vi "32 Channel Model.vi"() -> ()   [LabVIEW 2018]
uses:
  <vilib>/Instr/_visa.llb/VISA Set IO Buffer Mask.ctl
  <vilib>/Instr/_visa.llb/VISA Configure Serial Port (Instr).vi
  <vilib>/Analysis/NI_AAL_SigProc.lvlib
panel:
  out "Difference Index":i32
  out "max difference":dbl
  out "C0 max value":dbl
  out "C0 index position":i32
  out "time in sec":u32
  out "Channel 33":i16[](graph)
  out "Channel 32":i16[](graph)
  out "C4  max value":dbl
  out "Ch4 index position":i32
  out "Channel 8 max":i32
  out "DIFFERENCE":dbl[](array[numeric])
  in  "?":bool
  in  "Select Channel 2":T1(ring)
  in  "Select Channel":T1(ring)
  out "Locations 28":dbl[](array[numeric])
  out "Locations C29":dbl[](array[numeric])
  out "Locations C30":dbl[](array[numeric])
  out "Locations C31":dbl[](array[numeric])
  out "Locations C24":dbl[](array[numeric])
  out "Locations 25":dbl[](array[numeric])
  out "Locations C26":dbl[](array[numeric])
  out "Locations C27":dbl[](array[numeric])
  out "Locations C20":dbl[](array[numeric])
  out "Locations C21":dbl[](array[numeric])
  out "Locations C22":dbl[](array[numeric])
  out "Locations C23":dbl[](array[numeric])
  out "Locations C16":dbl[](array[numeric])
  out "Locations C17":dbl[](array[numeric])
  out "Locations C18":dbl[](array[numeric])
  out "Locations C19":dbl[](array[numeric])
  out "Locations 12":dbl[](array[numeric])
  out "Locations 13":dbl[](array[numeric])
  out "Locations C14":dbl[](array[numeric])
  out "Locations C15":dbl[](array[numeric])
  out "Locations C8":dbl[](array[numeric])
  out "Locations C9":dbl[](array[numeric])
  out "Locations C10":dbl[](array[numeric])
  out "Locations C11":dbl[](array[numeric])
  out "Locations C4":dbl[](array[numeric])
  out "Locations C5":dbl[](array[numeric])
  out "Locations C6":dbl[](array[numeric])
  out "Locations C7":dbl[](array[numeric])
  out "Locations C3":dbl[](array[numeric])
  out "Locations C2":dbl[](array[numeric])
  out "Locations C1":dbl[](array[numeric])
  out "Locations C0":dbl[](array[numeric])
  in  "Infinite":bool
  in  "Stimulate":bool
  in  "Value 4":dbl=3.0 min=-10.0 max=10.0 step=0.01
  in  "Time 4":dbl=0.003 min=0.0001 max=60.0 step=1e-06
  in  "# of Pulse \n  Cycles":u16=24 min=1 step=1
  in  "Time 3":dbl=0.003 min=0.0001 max=60.0 step=1e-06
  in  "Value 3":dbl=-3.0 min=-10.0 max=10.0 step=0.01
  in  "Time 2":dbl=0.003 min=0.0001 max=60.0 step=1e-06
  in  "Value 2":dbl min=-10.0 max=10.0 step=0.01
  in  "# of Stimulation\n       Cycles":u16=1 min=1 max=65534 step=1
  in  "Time":dbl=0.9 min=0.0001 max=60.0 step=1e-06
  in  "Value":dbl min=-10.0 max=10.0 step=0.01
  in  "Stop Stimulation":bool
  in  "Channel Number":u8=1 max=31 step=1
  out "C31":bool
  out "C30":bool
  out "C29":bool
  out "C28":bool
  out "C27":bool
  out "C26":bool
  out "C25":bool
  out "C24":bool
  out "C20":bool
  out "C21":bool
  out "C22":bool
  out "C23":bool
  out "C19":bool
  out "C18":bool
  out "C17":bool
  out "C16":bool
  out "C15":bool
  out "C14":bool
  out "C13":bool
  out "C12":bool
  out "C8":bool
  out "C9":bool
  out "C10":bool
  out "C11":bool
  out "C4":bool
  out "C5":bool
  out "C6":bool
  out "C7":bool
  out "C0":bool
  out "C1":bool
  out "C2":bool
  out "C3":bool
  in  "?":bool
  out "?":bool
  out "Channel 31":i16[](graph)
  out "Channel 30":i16[](graph)
  out "Channel 29":i16[](graph)
  out "C28":u16
  out "C29":u16
  out "C30":u16
  out "C31":u16
  out "Channel 28":i16[](graph)
  out "Channel 27":i16[](graph)
  out "Channel 26":i16[](graph)
  out "Channel 25":i16[](graph)
  out "C27":u16
  out "C26":u16
  out "C25":u16
  out "C24":u16
  out "Channel 23":i16[](graph)
  out "Channel 22":i16[](graph)
  out "Channel 21":i16[](graph)
  out "C23":u16
  out "C22":u16
  out "C21":u16
  out "C20":u16
  out "Channel 20":i16[](graph)
  out "Channel 19":i16[](graph)
  out "Channel 18":i16[](graph)
  out "Channel 17":i16[](graph)
  out "C19":u16
  out "C18":u16
  out "C17":u16
  out "C16":u16
  out "Channel 16":i16[](graph)
  out "Channel 15":i16[](graph)
  out "Channel 14":i16[](graph)
  out "Channel 13":i16[](graph)
  out "C15":u16
  out "C14":u16
  out "C13":u16
  out "C12":u16
  out "Channel 12":i16[](graph)
  out "Channel 24":i16[](graph)
  out "Channel 11":i16[](graph)
  out "Channel 10":i16[](graph)
  out "Channel 9":i16[](graph)
  out "C11":u16
  out "C10":u16
  out "C9":u16
  out "C8":u16
  out "Channel 8":i16[](graph)
  out "C7":u16
  out "Channel 7":i16[](graph)
  out "C6":u16
  out "Channel 6":i16[](graph)
  out "C5":u16
  out "Channel 5":i16[](graph)
  out "C4":u16
  out "Channel 4":i16(graph)
  out "Channel 3":i16(graph)
  out "C3":u16
  out "C2":u16
  out "Channel 2":i16(graph)
  out "C1":u16
  out "Channel 1":i16(graph)
  out "Channel 0":i16(graph)
  out "C0":u16
  out "Ring 7":bool
  out "Ring 6":bool
  out "Ring 5":bool
  out "Ring 4":bool
  out "Ring 3":bool
  out "Ring 2":bool
  out "Ring 1":bool
  out "Ring 0":bool
  in  "VISA Stationary Port":refnum<visa-resource-name>
  # "Ring 0"
  # "Ring 0"
  # "Ring 1"
  # "Ring 2"
  # "Ring 1"
  # "Ring 3"
  # "Ring 4"
  # "Ring 5"
  # "Ring 7"
  # "Ring 6"
  # "Ring 2"
  # "Ring 3"
  # "Ring 4"
  # "Ring 5"
  # "Ring 6"
  # "Ring 7"
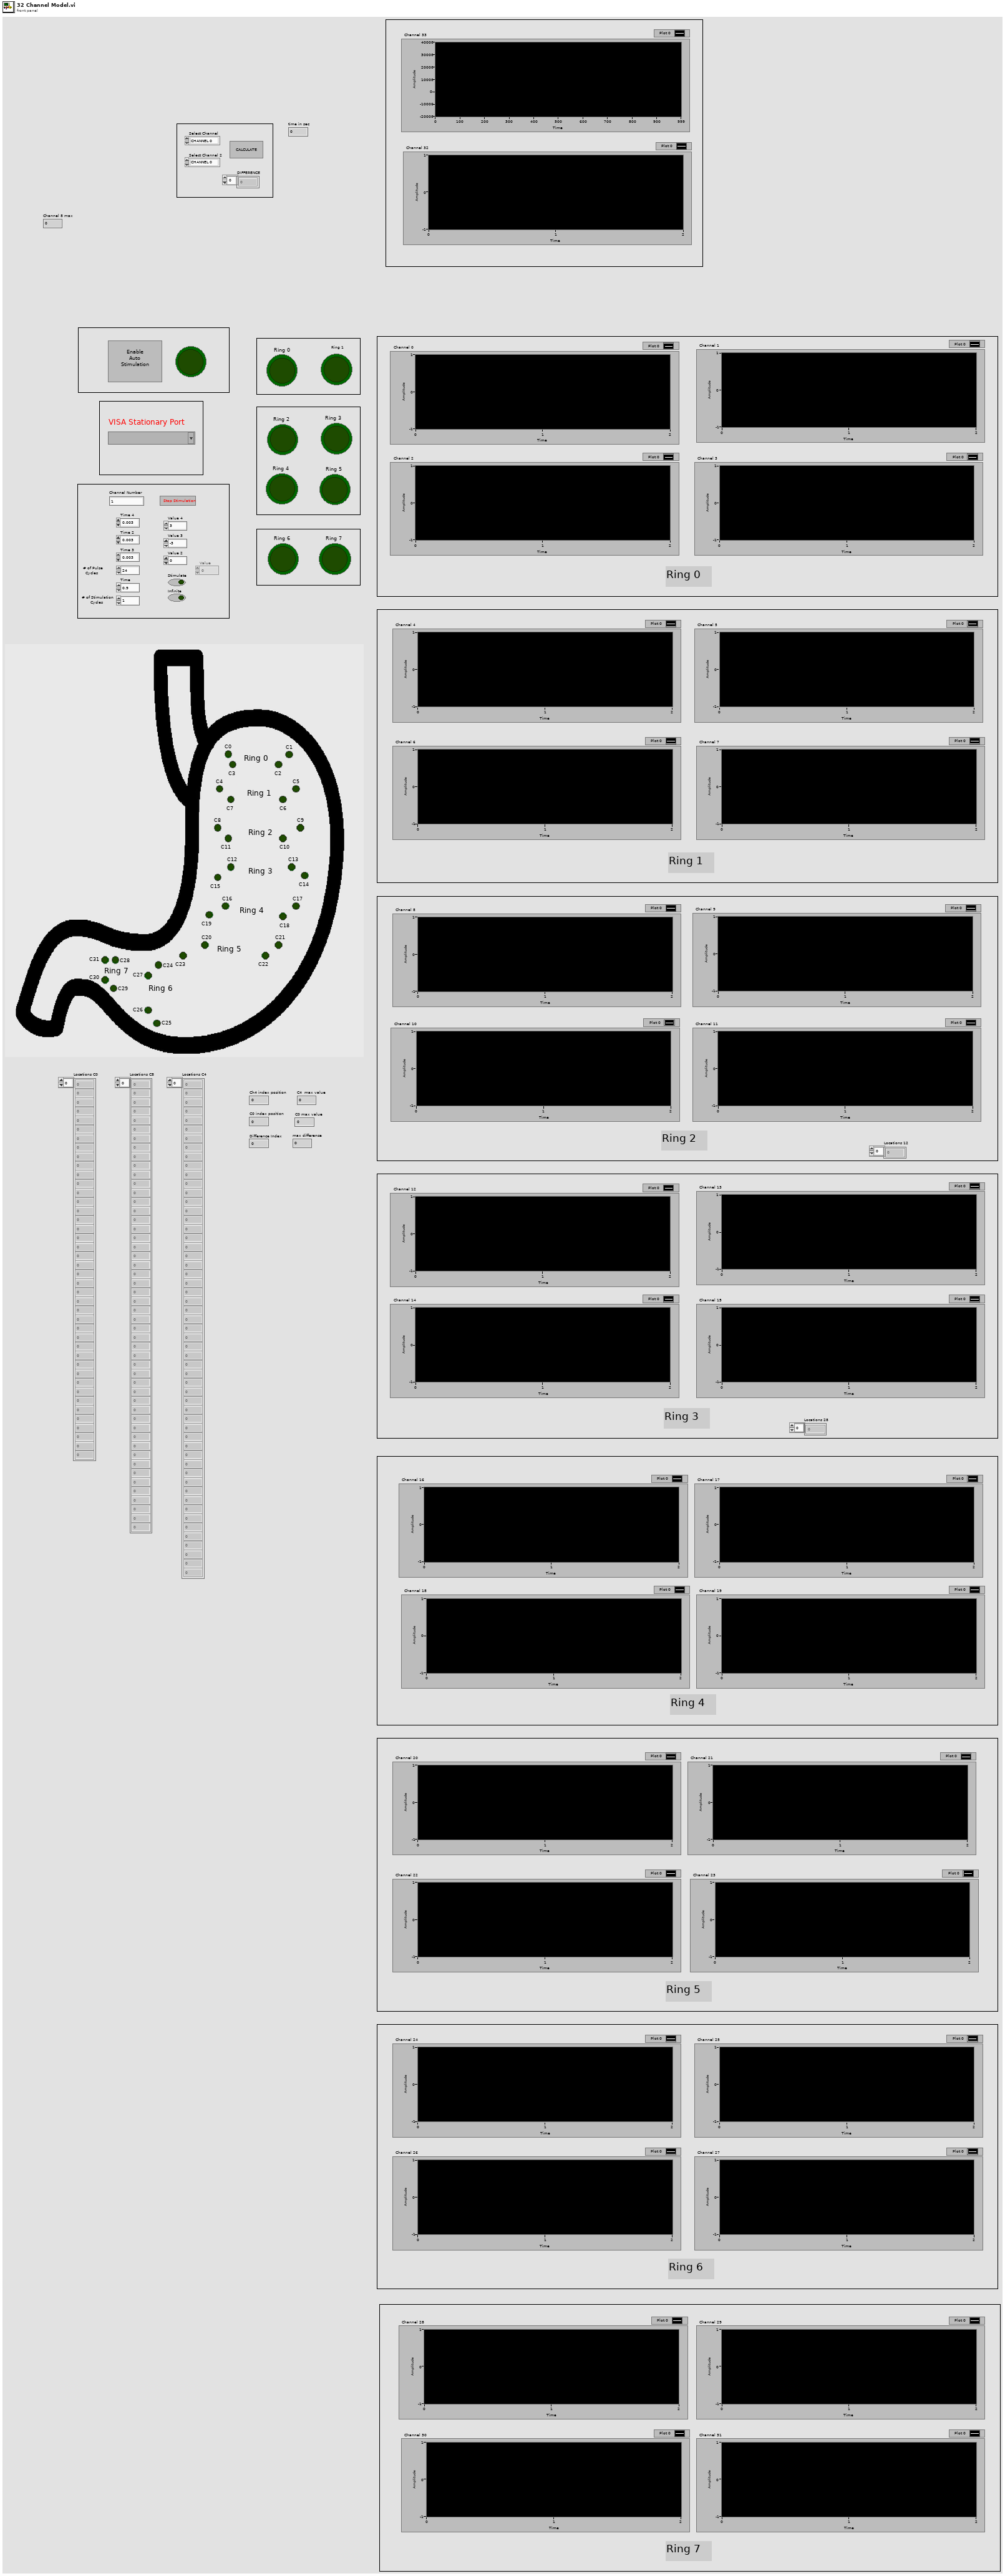
[diagram p1: front panel]
types:
  T1 = enum16{"CHANNEL 0", "CHANNEL 1", "CHANNEL 2 ", "CHANNEL 3 ", "CHANNEL 4 ", "CHANNEL 5 ", "CHANNEL 6", "CHANNEL  7", "CHANNEL 8 ", "CHANNEL 9", "CHANNEL 10", "CHANNEL 11", "CHANNEL 12", "CHANNEL 13", "CHANNEL 14", "CHANNEL 15", "CHANNEL 16", "CHANNEL 17", "CHANNEL 18", "CHANNEL 19", "CHANNEL 20", "CHANNEL 21", "CHANNEL 22", "CHANNEL 23", "CHANNEL 24", "CHANNEL 25", "CHANNEL 26", "CHANNEL 27", "CHANNEL 28", "CHANNEL 29", "CHANNEL 30", "CHANNEL 31"}
  T2 = typedef "VISA Set IO Buffer Mask.ctl" = u16
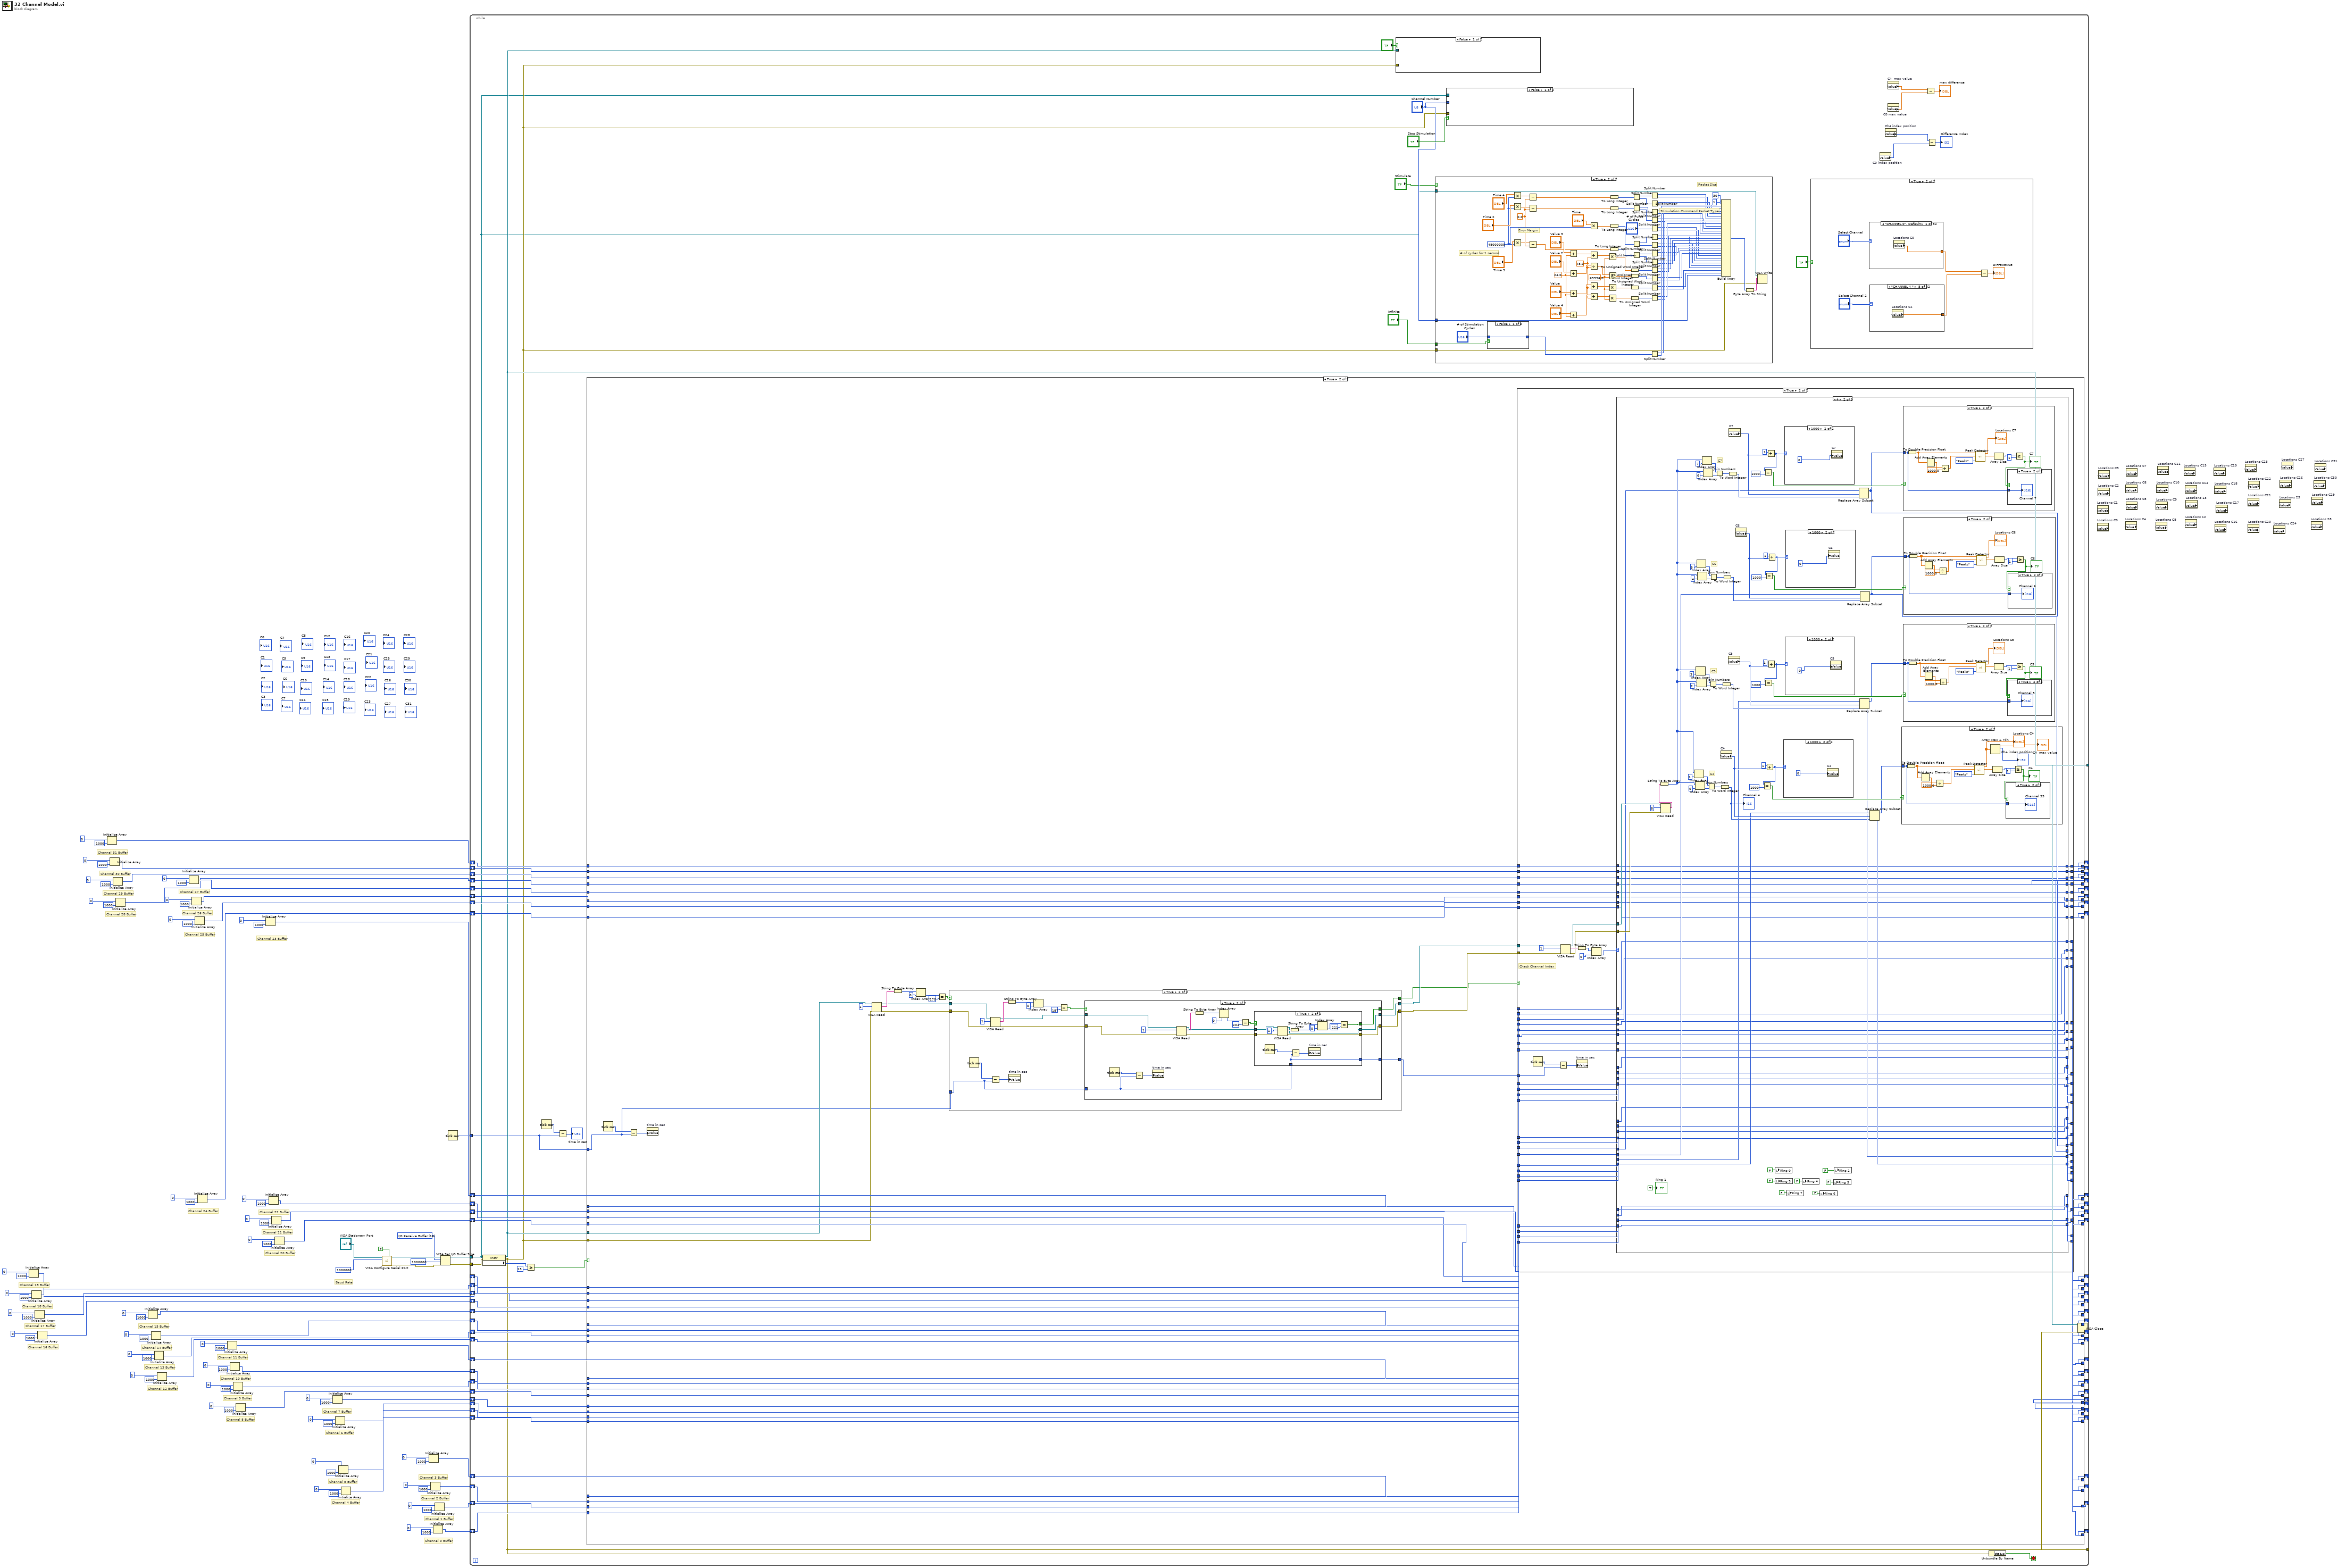
[diagram p0: block diagram]
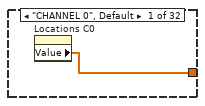
[diagram p3: hidden frame]
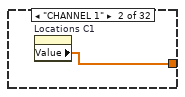
[diagram p4: hidden frame]
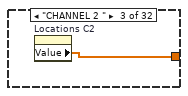
[diagram p5: hidden frame]
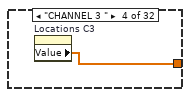
[diagram p6: hidden frame]
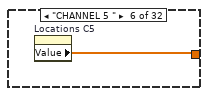
[diagram p7: hidden frame]
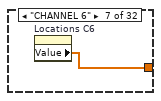
[diagram p8: hidden frame]
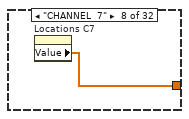
[diagram p9: hidden frame]
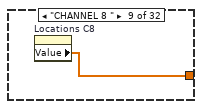
[diagram p10: hidden frame]
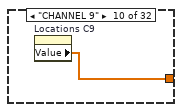
[diagram p11: hidden frame]
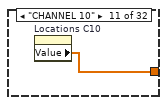
[diagram p12: hidden frame]
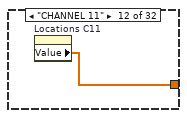
[diagram p13: hidden frame]
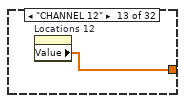
[diagram p14: hidden frame]
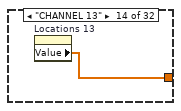
[diagram p15: hidden frame]
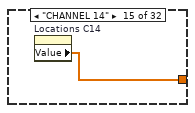
[diagram p16: hidden frame]
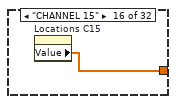
[diagram p17: hidden frame]
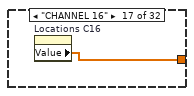
[diagram p18: hidden frame]
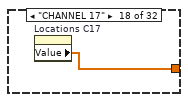
[diagram p19: hidden frame]
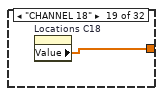
[diagram p20: hidden frame]
diagram:
  w104 = T2 16 items=["I/O Receive Buffer"=16, "I/O Transmit Buffer"=32, "I/O Receive and Transmit Buffer"=48] ("Mask")
  # "Channel 31 Buffer"
  # "Channel 30 Buffer"
  # "Channel 29 Buffer"
  # "Channel 28 Buffer"
  # "Channel 27 Buffer"
  # "Channel 26 Buffer"
  # "Channel 25 Buffer"
  # "Channel 24 Buffer"
  # "Channel 23 Buffer"
  # "Channel 22 Buffer"
  # "Channel 21 Buffer"
  # "Channel 20 Buffer"
  # "Channel 19 Buffer"
  # "Channel 18 Buffer"
  # "Channel 17 Buffer"
  # "Channel 16 Buffer"
  # "Channel 15 Buffer"
  # "Channel 14 Buffer"
  # "Channel 13 Buffer"
  # "Channel 12 Buffer"
  # "Channel 11 Buffer"
  # "Channel 10 Buffer"
  # "Channel 9 Buffer"
  # "Channel 8 Buffer"
  # "Channel 7 Buffer"
  # "Channel 6 Buffer"
  # "Channel 5 Buffer"
  # "Channel 4 Buffer"
  # "Channel 3 Buffer"
  # "Channel 2 Buffer"
  # "Channel 1 Buffer"
  # "Channel 0 Buffer"
  # "Baud Rate"
  n1 = Initialize Array(i16 0 ("element"), 1000 ("dimension size")) -> (w38:i16[])
  n2 = Initialize Array(i16 0 ("element"), 1000 ("dimension size")) -> (w39:i16[])
  n3 = Initialize Array(i16 0 ("element"), 1000 ("dimension size")) -> (w40:i16[])
  n4 = Initialize Array(i16 0 ("element"), 1000 ("dimension size")) -> (w41:i16[])
  n5 = Initialize Array(i16 0 ("element"), 1000 ("dimension size")) -> (w2:i16[])
  n6 = Initialize Array(i16 0 ("element"), 1000 ("dimension size")) -> (w3:i16[])
  n7 = Initialize Array(i16 0 ("element"), 1000 ("dimension size")) -> (w4:i16[])
  n8 = Initialize Array(i16 0 ("element"), 1000 ("dimension size")) -> (w5:i16[])
  n9 = Initialize Array(i16 0 ("element"), 1000 ("dimension size")) -> (w50:i16[])
  n10 = Initialize Array(i16 0 ("element"), 1000 ("dimension size")) -> (w51:i16[])
  n11 = Initialize Array(i16 0 ("element"), 1000 ("dimension size")) -> (w52:i16[])
  n12 = Initialize Array(i16 0 ("element"), 1000 ("dimension size")) -> (w53:i16[])
  n13 = Initialize Array(i16 0 ("element"), 1000 ("dimension size")) -> (w14:i16[])
  n14 = Initialize Array(i16 0 ("element"), 1000 ("dimension size")) -> (w15:i16[])
  n15 = Initialize Array(i16 0 ("element"), 1000 ("dimension size")) -> (w16:i16[])
  n16 = Initialize Array(i16 0 ("element"), 1000 ("dimension size")) -> (w17:i16[])
  n17 = Initialize Array(i16 0 ("element"), 1000 ("dimension size")) -> (w62:i16[])
  n18 = Initialize Array(i16 0 ("element"), 1000 ("dimension size")) -> (w63:i16[])
  n19 = Initialize Array(i16 0 ("element"), 1000 ("dimension size")) -> (w64:i16[])
  n20 = Initialize Array(i16 0 ("element"), 1000 ("dimension size")) -> (w65:i16[])
  n21 = Initialize Array(i16 0 ("element"), 1000 ("dimension size")) -> (w26:i16[])
  n22 = Initialize Array(i16 0 ("element"), 1000 ("dimension size")) -> (w27:i16[])
  n23 = Initialize Array(i16 0 ("element"), 1000 ("dimension size")) -> (w28:i16[])
  n24 = Initialize Array(i16 0 ("element"), 1000 ("dimension size")) -> (w29:i16[])
  n25 = Initialize Array(i16 0 ("element"), 1000 ("dimension size")) -> (w74:i16[])
  n26 = Initialize Array(i16 0 ("element"), 1000 ("dimension size")) -> (w75:i16[])
  n27 = Initialize Array(i16 0 ("element"), 1000 ("dimension size")) -> (w76:i16[])
  n28 = Initialize Array(i16 0 ("element"), 1000 ("dimension size")) -> (w77:i16[])
  n29 = call-poly "VISA Configure Serial Port"("VISA resource name"="VISA Stationary Port", "Enable Termination\nChar (T)"=FALSE ("Enable Termination\nChar (T)"), "baud rate (9600)"=u32 1000000) -> ("VISA resource name out"=w105:refnum<visa-resource-name>, "error out"=w102:errorcluster)  [unwired: 11 in]
  n30 = Initialize Array(i16 0 ("element"), 1000 ("dimension size")) -> (w86:i16[])
  n31 = Initialize Array(i16 0 ("element"), 1000 ("dimension size")) -> (w89:i16[])
  n32 = Initialize Array(i16 0 ("element"), 1000 ("dimension size")) -> (w95:i16[])
  n33 = Initialize Array(i16 0 ("element"), 1000 ("dimension size")) -> (w92:i16[])
  n34 = VISA Set I/O Buffer Size(VISA resource name=w105, mask (16)=w104, size (4096)=u32 1000000, error in (no error)=w102) -> (VISA resource name out=w101:refnum<visa-resource-name>, error out=w100:errorcluster)
  n35 = Tick Count (ms)() -> (millisecond timer value=w1:u32)
  n36 = while {
    tunnel: w101 -> [w119]
    tunnel: w100 -> [w195]
    tunnel: [w126] -> w99
    tunnel: [w120] -> w98
    shift-right: [w189] -> _
    shift-left: w95 -> [w190]
    shift-right: [w187] -> _
    shift-left: w92 -> [w188]
    shift-right: [w185] -> _
    shift-left: w89 -> [w186]
    shift-right: [w183] -> _
    shift-left: w86 -> [w184]
    shift-right: [w178] -> _
    shift-left: w77 -> [w182]
    shift-right: [w177] -> _
    shift-left: w76 -> [w181]
    shift-right: [w176] -> _
    shift-left: w75 -> [w180]
    shift-right: [w175] -> _
    shift-left: w74 -> [w179]
    shift-right: [w170] -> _
    shift-left: w65 -> [w174]
    shift-right: [w169] -> _
    shift-left: w64 -> [w173]
    shift-right: [w168] -> _
    shift-left: w63 -> [w172]
    shift-right: [w167] -> _
    shift-left: w62 -> [w171]
    shift-right: [w159] -> _
    shift-left: w53 -> [w166]
    shift-right: [w160] -> _
    shift-left: w52 -> [w165]
    shift-right: [w161] -> _
    shift-left: w51 -> [w164]
    shift-right: [w162] -> _
    shift-left: w50 -> [w163]
    shift-right: [w154] -> _
    shift-left: w41 -> [w158]
    shift-right: [w153] -> _
    shift-left: w40 -> [w157]
    shift-right: [w152] -> _
    shift-left: w39 -> [w156]
    shift-right: [w151] -> _
    shift-left: w38 -> [w155]
    shift-right: [w146] -> _
    shift-left: w29 -> [w150]
    shift-right: [w145] -> _
    shift-left: w28 -> [w149]
    shift-right: [w144] -> _
    shift-left: w27 -> [w148]
    shift-right: [w143] -> _
    shift-left: w26 -> [w147]
    shift-right: [w138] -> _
    shift-left: w17 -> [w142]
    shift-right: [w137] -> _
    shift-left: w16 -> [w141]
    shift-right: [w136] -> _
    shift-left: w15 -> [w140]
    shift-right: [w135] -> _
    shift-left: w14 -> [w139]
    shift-right: [w134] -> _
    shift-left: w5 -> [w133]
    shift-right: [w129] -> _
    shift-left: w4 -> [w132]
    shift-right: [w128] -> _
    shift-left: w3 -> [w131]
    shift-right: [w127] -> _
    shift-left: w2 -> [w130]
    tunnel: w1 -> [w116]
    stop <- w191 stop-if-true
    n37 = property class="Instr"(reference=w119, error in=w195) -> (reference out=w126:refnum<visa-resource-name>, error out=w120:errorcluster, "Serial Settings:Number of Bytes at Serial Port"=w194:u32)
    n38 = Greater Or Equal?(x=w194, y=u32 13) -> (x >= y?=w192:bool)
    n39 = Tick Count (ms)() -> (millisecond timer value=w117:u32)
    n40 = Subtract(x=w117, y=w116) -> (x-y=→"time in sec":u32)
    n41 = case shown="True" w192 {
      tunnel: w126 -> [_ w414]
      tunnel: w120 -> [_ w413]
      tunnel: w190 -> [w399 w481]
      tunnel: [w399 w480] -> w189
      tunnel: w188 -> [w398 w479]
      tunnel: [w398 w478] -> w187
      tunnel: w186 -> [w397 w477]
      tunnel: [w397 w476] -> w185
      tunnel: w184 -> [w396 w475]
      tunnel: [w396 w474] -> w183
      tunnel: w182 -> [w395 w473]
      tunnel: w181 -> [w394 w472]
      tunnel: w180 -> [w393 w471]
      tunnel: w179 -> [w392 w470]
      tunnel: [w395 w469] -> w178
      tunnel: [w394 w468] -> w177
      tunnel: [w393 w467] -> w176
      tunnel: [w392 w466] -> w175
      tunnel: w174 -> [w391 w465]
      tunnel: w173 -> [w390 w464]
      tunnel: w172 -> [w389 w463]
      tunnel: w171 -> [w388 w462]
      tunnel: [w391 w461] -> w170
      tunnel: [w390 w460] -> w169
      tunnel: [w389 w459] -> w168
      tunnel: [w388 w458] -> w167
      tunnel: w166 -> [w387 w457]
      tunnel: w165 -> [w386 w456]
      tunnel: w164 -> [w385 w455]
      tunnel: w163 -> [w384 w454]
      tunnel: [w384 w453] -> w162
      tunnel: [w385 w452] -> w161
      tunnel: [w386 w451] -> w160
      tunnel: [w387 w450] -> w159
      tunnel: w158 -> [w383 w446]
      tunnel: w157 -> [w382 w447]
      tunnel: w156 -> [w381 w448]
      tunnel: w155 -> [w380 w449]
      tunnel: [w383 w445] -> w154
      tunnel: [w382 w444] -> w153
      tunnel: [w381 w443] -> w152
      tunnel: [w380 w442] -> w151
      tunnel: w150 -> [w379 w441]
      tunnel: w149 -> [w378 w440]
      tunnel: w148 -> [w377 w439]
      tunnel: w147 -> [w376 w438]
      tunnel: [w379 w437] -> w146
      tunnel: [w378 w436] -> w145
      tunnel: [w377 w435] -> w144
      tunnel: [w376 w434] -> w143
      tunnel: w142 -> [w375 w433]
      tunnel: w141 -> [w374 w432]
      tunnel: w140 -> [w373 w431]
      tunnel: w139 -> [w372 w430]
      tunnel: [w375 w429] -> w138
      tunnel: [w374 w428] -> w137
      tunnel: [w373 w427] -> w136
      tunnel: [w372 w426] -> w135
      tunnel: [w371 w425] -> w134
      tunnel: w133 -> [w371 w424]
      tunnel: w132 -> [w370 w423]
      tunnel: w131 -> [w369 w422]
      tunnel: w130 -> [w368 w421]
      tunnel: [w370 w420] -> w129
      tunnel: [w369 w419] -> w128
      tunnel: [w368 w418] -> w127
      tunnel: w116 -> [_ w401]
      frame False {
      }
      frame True {
        n42 = Tick Count (ms)() -> (millisecond timer value=w403:u32)
        n43 = Subtract(x=w403, y=w401) -> (x-y=w402:u32)
        n44 = property on="time in sec" class="DigNum (strict)"("Value"=w402) -> ()  [unwired: 2 in, 2 out]
        n45 = VISA Read(VISA resource name=w414, byte count=u32 1, error in (no error)=w413) -> (VISA resource name out=w405:refnum<visa-resource-name>, read buffer=w411:string, error out=w404:errorcluster)  [unwired: 1 out]
        n46 = String To Byte Array(string=w411) -> (unsigned byte array=w410:u8[])
        n47 = Index Array(array=w410, index=0) -> (element=w408:u8)
        n48 = Equal?(x=w408, y=u8 170) -> (x = y?=w406:bool)
        n49 = case shown="True" w406 {
          tunnel: w405 -> [w486 w498]
          tunnel: w404 -> [w487 w497]
          tunnel: [FALSE w494] -> w415
          tunnel: [w486 w493] -> w417
          tunnel: [w487 w492] -> w416
          tunnel: w401 -> [w482 w489]
          tunnel: [w482 w488] -> w400
          frame False {
            n50 = Tick Count (ms)() -> (millisecond timer value=w483:u32)
            n51 = Subtract(x=w483, y=w482) -> (x-y=w484:u32)
            n52 = property on="time in sec" class="DigNum (strict)"("Value"=w484) -> ()  [unwired: 2 in, 2 out]
          }
          frame True {
            n53 = Tick Count (ms)() -> (millisecond timer value=w490:u32)
            n54 = VISA Read(VISA resource name=w498, byte count=u32 1, error in (no error)=w497) -> (VISA resource name out=w496:refnum<visa-resource-name>, read buffer=w504:string, error out=w495:errorcluster)  [unwired: 1 out]
            n55 = Subtract(x=w490, y=w489) -> (x-y=w491:u32)
            n56 = String To Byte Array(string=w504) -> (unsigned byte array=w503:u8[])
            n57 = property on="time in sec" class="DigNum (strict)"("Value"=w491) -> ()  [unwired: 2 in, 2 out]
            n58 = Index Array(array=w503, index=0) -> (element=w501:u8)
            n59 = Equal?(x=w501, y=u8 187) -> (x = y?=w499:bool)
            n60 = case shown="True" w499 {
              tunnel: w496 -> [w510 w523]
              tunnel: w495 -> [w509 w522]
              tunnel: [FALSE w518] -> w494
              tunnel: [w510 w517] -> w493
              tunnel: [w509 w516] -> w492
              tunnel: w489 -> [w506 w513]
              tunnel: [w506 w512] -> w488
              frame False {
                n61 = Tick Count (ms)() -> (millisecond timer value=w507:u32)
                n62 = Subtract(x=w507, y=w506) -> (x-y=w508:u32)
                n63 = property on="time in sec" class="DigNum (strict)"("Value"=w508) -> ()  [unwired: 2 in, 2 out]
              }
              frame True {
                n64 = Tick Count (ms)() -> (millisecond timer value=w514:u32)
                n65 = Subtract(x=w514, y=w513) -> (x-y=w515:u32)
                n66 = property on="time in sec" class="DigNum (strict)"("Value"=w515) -> ()  [unwired: 2 in, 2 out]
                n67 = VISA Read(VISA resource name=w523, byte count=u32 1, error in (no error)=w522) -> (VISA resource name out=w521:refnum<visa-resource-name>, read buffer=w528:string, error out=w520:errorcluster)  [unwired: 1 out]
                n68 = String To Byte Array(string=w528) -> (unsigned byte array=w527:u8[])
                n69 = Index Array(array=w527, index=0) -> (element=w525:u8)
                n70 = Equal?(x=w525, y=u8 204) -> (x = y?=w519:bool)
                n71 = case shown="True" w519 {
                  tunnel: w521 -> [w533 w543]
                  tunnel: w520 -> [w534 w542]
                  tunnel: [FALSE w541] -> w518
                  tunnel: [w533 w540] -> w517
                  tunnel: [w534 w539] -> w516
                  tunnel: w513 -> [w530 w536]
                  tunnel: [w530 w536] -> w512
                  frame False {
                    n72 = Tick Count (ms)() -> (millisecond timer value=w531:u32)
                    n73 = Subtract(x=w531, y=w530) -> (x-y=w532:u32)
                    n74 = property on="time in sec" class="DigNum (strict)"("Value"=w532) -> ()  [unwired: 2 in, 2 out]
                  }
                  frame True {
                    n75 = Tick Count (ms)() -> (millisecond timer value=w537:u32)
                    n76 = VISA Read(VISA resource name=w543, byte count=u32 1, error in (no error)=w542) -> (VISA resource name out=w540:refnum<visa-resource-name>, read buffer=w548:string, error out=w539:errorcluster)  [unwired: 1 out]
                    n77 = String To Byte Array(string=w548) -> (unsigned byte array=w547:u8[])
                    n78 = Subtract(x=w537, y=w536) -> (x-y=w538:u32)
                    n79 = property on="time in sec" class="DigNum (strict)"("Value"=w538) -> ()  [unwired: 2 in, 2 out]
                    n80 = Index Array(array=w547, index=0) -> (element=w545:u8)
                    n81 = Equal?(x=w545, y=u8 221) -> (x = y?=w541:bool)
                  }
                }
              }
            }
          }
        }
        n82 = case shown="True" w415 {
          tunnel: w417 -> [_ w657]
          tunnel: w416 -> [_ w656]
          tunnel: w481 -> [w581 w648]
          tunnel: [w581 w647] -> w480
          tunnel: w479 -> [w580 w645]
          tunnel: [w580 w646] -> w478
          tunnel: w477 -> [w579 w644]
          tunnel: [w579 w643] -> w476
          tunnel: w475 -> [w578 w642]
          tunnel: [w578 w641] -> w474
          tunnel: w473 -> [w577 w640]
          tunnel: w472 -> [w576 w639]
          tunnel: w471 -> [w575 w638]
          tunnel: w470 -> [w574 w637]
          tunnel: [w577 w636] -> w469
          tunnel: [w576 w635] -> w468
          tunnel: [w575 w634] -> w467
          tunnel: [w574 w633] -> w466
          tunnel: w465 -> [w573 w631]
          tunnel: w464 -> [w572 w632]
          tunnel: w463 -> [w570 w630]
          tunnel: w462 -> [w571 w629]
          tunnel: [w573 w628] -> w461
          tunnel: [w572 w627] -> w460
          tunnel: [w570 w626] -> w459
          tunnel: [w571 w625] -> w458
          tunnel: w457 -> [w569 w624]
          tunnel: w456 -> [w568 w623]
          tunnel: w455 -> [w567 w622]
          tunnel: w454 -> [w566 w621]
          tunnel: [w566 w620] -> w453
          tunnel: [w567 w619] -> w452
          tunnel: [w568 w618] -> w451
          tunnel: [w569 w617] -> w450
          tunnel: w449 -> [w562 w616]
          tunnel: w448 -> [w563 w615]
          tunnel: w447 -> [w564 w614]
          tunnel: w446 -> [w565 w613]
          tunnel: [w565 w612] -> w445
          tunnel: [w564 w611] -> w444
          tunnel: [w563 w610] -> w443
          tunnel: [w562 w609] -> w442
          tunnel: w441 -> [w561 w608]
          tunnel: w440 -> [w560 w607]
          tunnel: w439 -> [w559 w606]
          tunnel: w438 -> [w558 w605]
          tunnel: [w561 w604] -> w437
          tunnel: [w560 w603] -> w436
          tunnel: [w559 w602] -> w435
          tunnel: [w558 w601] -> w434
          tunnel: w433 -> [w557 w600]
          tunnel: w432 -> [w556 w599]
          tunnel: w431 -> [w555 w598]
          tunnel: w430 -> [w554 w597]
          tunnel: [w557 w596] -> w429
          tunnel: [w556 w595] -> w428
          tunnel: [w555 w594] -> w427
          tunnel: [w554 w593] -> w426
          tunnel: [w553 w592] -> w425
          tunnel: w424 -> [w553 w591]
          tunnel: w423 -> [w552 w590]
          tunnel: w422 -> [w551 w589]
          tunnel: w421 -> [w550 w588]
          tunnel: [w552 w587] -> w420
          tunnel: [w551 w586] -> w419
          tunnel: [w550 w585] -> w418
          tunnel: w400 -> [_ w582]
          frame False {
          }
          frame True {
            # "Check Channel Index"
            n83 = Tick Count (ms)() -> (millisecond timer value=w583:u32)
            n84 = Subtract(x=w583, y=w582) -> (x-y=w584:u32)
            n85 = VISA Read(VISA resource name=w657, byte count=u32 1, error in (no error)=w656) -> (VISA resource name out=w650:refnum<visa-resource-name>, read buffer=w654:string, error out=w649:errorcluster)  [unwired: 1 out]
            n86 = property on="time in sec" class="DigNum (strict)"("Value"=w584) -> ()  [unwired: 2 in, 2 out]
            n87 = String To Byte Array(string=w654) -> (unsigned byte array=w652:u8[])
            n88 = Index Array(array=w652, index=0) -> (element=w651:u8)
            n89 = case shown="4" w651 {
              tunnel: w650 -> [w750 w897 w1048 w1198 w1347 w1496 w1645 w1794 _]
              tunnel: w649 -> [w749 w896 w1047 w1197 w1346 w1495 w1644 w1793 _]
              tunnel: w648 -> [w736 w894 w1045 w1195 w1344 w1493 w1642 w1792 w1883]
              tunnel: [w662 w894 w1045 w1195 w1344 w1493 w1642 w1792 w1883] -> w647
              tunnel: [w725 w893 w1044 w1194 w1343 w1492 w1641 w1791 w1882] -> w646
              tunnel: w645 -> [w715 w893 w1044 w1194 w1343 w1492 w1641 w1791 w1882]
              tunnel: w644 -> [w713 w892 w1043 w1193 w1342 w1491 w1640 w1790 w1881]
              tunnel: [w712 w892 w1043 w1193 w1342 w1491 w1640 w1790 w1881] -> w643
              tunnel: w642 -> [w702 w891 w1042 w1192 w1341 w1490 w1639 w1789 w1880]
              tunnel: [w701 w891 w1042 w1192 w1341 w1490 w1639 w1789 w1880] -> w641
              tunnel: w640 -> [w699 w847 w1041 w1191 w1340 w1489 w1638 w1788 w1879]
              tunnel: w639 -> [w698 w846 w1040 w1190 w1339 w1488 w1637 w1787 w1878]
              tunnel: w638 -> [w697 w845 w1039 w1189 w1338 w1487 w1636 w1786 w1877]
              tunnel: w637 -> [w696 w844 w1038 w1188 w1337 w1486 w1635 w1785 w1876]
              tunnel: [w699 w843 w1041 w1191 w1340 w1489 w1638 w1788 w1879] -> w636
              tunnel: [w698 w842 w1040 w1190 w1339 w1488 w1637 w1787 w1878] -> w635
              tunnel: [w697 w841 w1039 w1189 w1338 w1487 w1636 w1786 w1877] -> w634
              tunnel: [w696 w840 w1038 w1188 w1337 w1486 w1635 w1785 w1876] -> w633
              tunnel: w632 -> [w693 w837 w991 w1186 w1335 w1484 w1633 w1783 w1874]
              tunnel: w631 -> [w694 w838 w992 w1187 w1336 w1485 w1634 w1784 w1875]
              tunnel: w630 -> [w692 w836 w990 w1185 w1334 w1483 w1632 w1782 w1873]
              tunnel: w629 -> [w691 w835 w989 w1184 w1333 w1482 w1631 w1781 w1872]
              tunnel: [w694 w838 w988 w1187 w1336 w1485 w1634 w1784 w1875] -> w628
              tunnel: [w693 w837 w987 w1186 w1335 w1484 w1633 w1783 w1874] -> w627
              tunnel: [w692 w836 w986 w1185 w1334 w1483 w1632 w1782 w1873] -> w626
              tunnel: [w691 w835 w985 w1184 w1333 w1482 w1631 w1781 w1872] -> w625
              tunnel: w624 -> [w690 w834 w984 w1135 w1332 w1481 w1620 w1780 w1871]
              tunnel: w623 -> [w689 w833 w983 w1136 w1331 w1480 w1619 w1779 w1870]
              tunnel: w622 -> [w687 w832 w982 w1137 w1330 w1479 w1618 w1778 w1869]
              tunnel: w621 -> [w688 w831 w981 w1138 w1329 w1478 w1617 w1777 w1868]
              tunnel: [w688 w831 w981 w1131 w1329 w1478 w1617 w1777 w1868] -> w620
              tunnel: [w687 w832 w982 w1132 w1330 w1479 w1618 w1778 w1869] -> w619
              tunnel: [w689 w833 w983 w1133 w1331 w1480 w1619 w1779 w1870] -> w618
              tunnel: [w690 w834 w984 w1134 w1332 w1481 w1620 w1780 w1871] -> w617
              tunnel: w616 -> [w683 w827 w977 w1127 w1276 w1474 w1613 w1773 w1864]
              tunnel: w615 -> [w684 w828 w978 w1128 w1277 w1475 w1614 w1774 w1865]
              tunnel: w614 -> [w685 w829 w979 w1129 w1278 w1476 w1615 w1775 w1866]
              tunnel: w613 -> [w686 w830 w980 w1130 w1279 w1477 w1616 w1776 w1867]
              tunnel: [w686 w830 w980 w1130 w1283 w1477 w1616 w1776 w1867] -> w612
              tunnel: [w685 w829 w979 w1129 w1282 w1476 w1615 w1775 w1866] -> w611
              tunnel: [w684 w828 w978 w1128 w1281 w1475 w1614 w1774 w1865] -> w610
              tunnel: [w683 w827 w977 w1127 w1280 w1474 w1613 w1773 w1864] -> w609
              tunnel: w608 -> [w682 w826 w976 w1126 w1275 w1424 w1612 w1772 w1863]
              tunnel: w607 -> [w681 w825 w975 w1125 w1274 w1423 w1611 w1771 w1862]
              tunnel: w606 -> [w680 w824 w974 w1124 w1273 w1422 w1610 w1770 w1861]
              tunnel: w605 -> [w679 w823 w973 w1123 w1272 w1421 w1609 w1769 w1860]
              tunnel: [w682 w826 w976 w1126 w1275 w1428 w1612 w1772 w1863] -> w604
              tunnel: [w681 w825 w975 w1125 w1274 w1427 w1611 w1771 w1862] -> w603
              tunnel: [w680 w824 w974 w1124 w1273 w1426 w1610 w1770 w1861] -> w602
              tunnel: [w679 w823 w973 w1123 w1272 w1425 w1609 w1769 w1860] -> w601
              tunnel: w600 -> [w678 w822 w972 w1122 w1271 w1420 w1569 w1768 w1859]
              tunnel: w599 -> [w677 w821 w971 w1121 w1270 w1419 w1568 w1767 w1858]
              tunnel: w598 -> [w676 w820 w970 w1120 w1269 w1418 w1567 w1766 w1857]
              tunnel: w597 -> [w675 w819 w969 w1119 w1268 w1417 w1566 w1765 w1856]
              tunnel: [w678 w822 w972 w1122 w1271 w1420 w1573 w1768 w1859] -> w596
              tunnel: [w677 w821 w971 w1121 w1270 w1419 w1572 w1767 w1858] -> w595
              tunnel: [w676 w820 w970 w1120 w1269 w1418 w1571 w1766 w1857] -> w594
              tunnel: [w675 w819 w969 w1119 w1268 w1417 w1570 w1765 w1856] -> w593
              tunnel: [w674 w818 w968 w1118 w1267 w1416 w1565 w1753 w1855] -> w592
              tunnel: w591 -> [w674 w818 w968 w1118 w1267 w1416 w1565 w1717 w1855]
              tunnel: w590 -> [w673 w817 w967 w1117 w1266 w1415 w1564 w1716 w1854]
              tunnel: w589 -> [w672 w816 w966 w1116 w1265 w1414 w1563 w1714 w1853]
              tunnel: w588 -> [w671 w815 w965 w1115 w1264 w1413 w1562 w1711 w1852]
              tunnel: [w673 w817 w967 w1117 w1266 w1415 w1564 w1715 w1854] -> w587
              tunnel: [w672 w816 w966 w1116 w1265 w1414 w1563 w1713 w1853] -> w586
              tunnel: [w671 w815 w965 w1115 w1264 w1413 w1562 w1712 w1852] -> w585
              frame 0 {
                # "C3"
                # "C2"
                # "C1"
                # "C0"
                n90 = VISA Read(VISA resource name=w750, byte count=u32 8, error in (no error)=w749) -> (read buffer=w747:string)  [unwired: 3 out]
                n91 = String To Byte Array(string=w747) -> (unsigned byte array=w700:u8[])
                n92 = Index Array(array=w700, index=1) -> (element=w746:u8)
                n93 = Index Array(array=w700, index=5) -> (element=w724:u8)
                n94 = Index Array(array=w700, index=3) -> (element=w727:u8)
                n95 = Index Array(array=w700, index=0) -> (element=w744:u8)
                n96 = Index Array(array=w700, index=4) -> (element=w722:u8)
                n97 = Index Array(array=w700, index=2) -> (element=w729:u8)
                n98 = Index Array(array=w700, index=7) -> (element=w703:u8)
                n99 = Index Array(array=w700, index=6) -> (element=w705:u8)
                n100 = Join Numbers(hi=w746, lo=w744) -> ((hi.lo)=w742:u16)
                n101 = Join Numbers(hi=w724, lo=w722) -> ((hi.lo)=w720:u16)
                n102 = Join Numbers(hi=w727, lo=w729) -> ((hi.lo)=w731:u16)
                n103 = Join Numbers(hi=w703, lo=w705) -> ((hi.lo)=w707:u16)
                n104 = property on="C1" class="DigNum (strict)"() -> ("Value"=w726:u16)  [unwired: 2 in, 2 out]
                n105 = property on="C0" class="DigNum (strict)"() -> ("Value"=w738:u16)  [unwired: 2 in, 2 out]
                n106 = property on="C3" class="DigNum (strict)"() -> ("Value"=w695:u16)  [unwired: 2 in, 2 out]
                n107 = To Word Integer(number=w742) -> (16bit integer=w661:i16)
                "Channel 0" <- w661
                n108 = property on="C2" class="DigNum (strict)"() -> ("Value"=w714:u16)  [unwired: 2 in, 2 out]
                n109 = To Word Integer(number=w720) -> (16bit integer=w659:i16)
                "Channel 2" <- w659
                n110 = To Word Integer(number=w731) -> (16bit integer=w660:i16)
                "Channel 1" <- w660
                n111 = To Word Integer(number=w707) -> (16bit integer=w658:i16)
                "Channel 3" <- w658
                n112 = Replace Array Subset(array=w736, new element=w661, index=w738) -> (w662:i16[])
                n113 = Replace Array Subset(array=w713, new element=w659, index=w714) -> (w712:i16[])
                n114 = Replace Array Subset(array=w715, new element=w660, index=w726) -> (w725:i16[])
                n115 = Replace Array Subset(array=w702, new element=w658, index=w695) -> (w701:i16[])
                n116 = Add(x=u16 1, y=w738) -> (x+y=w740:u16)
                n117 = Equal?(x=w740, y=u16 1000) -> (x = y?=w737:bool)
                n118 = Add(x=u16 1, y=w714) -> (x+y=w718:u16)
                n119 = Equal?(x=w718, y=u16 1000) -> (x = y?=w716:bool)
                n120 = Add(x=u16 1, y=w726) -> (x+y=w733:u16)
                n121 = Equal?(x=w733, y=u16 1000) -> (x = y?=w735:bool)
                n122 = Add(x=u16 1, y=w695) -> (x+y=w709:u16)
                n123 = Equal?(x=w709, y=u16 1000) -> (x = y?=w711:bool)
                n124 = local write "Ring 3"(FALSE ("Ring 0")) -> ()
                n125 = case shown="1000" w740 {
                  selector: w740 -> [w804 _]
                  frame 0, Default {
                    n126 = property on="C0" class="DigNum (strict)"("Value"=w804) -> ()  [unwired: 2 in, 2 out]
                  }
                  frame 1000 {
                    n127 = property on="C0" class="DigNum (strict)"("Value"=0) -> ()  [unwired: 2 in, 2 out]
                  }
                }
                n128 = case shown="1000" w718 {
                  selector: w718 -> [w775 _]
                  frame 0, Default {
                    n129 = property on="C2" class="DigNum (strict)"("Value"=w775) -> ()  [unwired: 2 in, 2 out]
                  }
                  frame 1000 {
                    n130 = property on="C2" class="DigNum (strict)"("Value"=0) -> ()  [unwired: 2 in, 2 out]
                  }
                }
                n131 = case shown="1000" w733 {
                  selector: w733 -> [w788 _]
                  frame 0, Default {
                    n132 = property on="C1" class="DigNum (strict)"("Value"=w788) -> ()  [unwired: 2 in, 2 out]
                  }
                  frame 1000 {
                    n133 = property on="C1" class="DigNum (strict)"("Value"=0) -> ()  [unwired: 2 in, 2 out]
                  }
                }
                n134 = local write "Ring 7"(FALSE ("Ring 0")) -> ()
                n135 = case shown="1000" w709 {
                  selector: w709 -> [w762 _]
                  frame 0, Default {
                    n136 = property on="C3" class="DigNum (strict)"("Value"=w762) -> ()  [unwired: 2 in, 2 out]
                  }
                  frame 1000 {
                    n137 = property on="C3" class="DigNum (strict)"("Value"=0) -> ()  [unwired: 2 in, 2 out]
                  }
                }
                n138 = local write "Ring 4"(FALSE ("Ring 0")) -> ()
                n139 = local write "Ring 1"(FALSE ("Ring 0")) -> ()
                n140 = local write "Ring 6"(FALSE ("Ring 0")) -> ()
                n141 = local write "Ring 5"(FALSE ("Ring 0")) -> ()
                n142 = local write "Ring 2"(FALSE ("Ring 0")) -> ()
                n143 = case shown="True" w711 {
                  tunnel: w701 -> [_ w756]
                  frame False {
                  }
                  frame True {
                    n144 = To Double Precision Float(number=w756) -> (double precision float=w752:dbl[])
                    n145 = Add Array Elements(numeric array=w752) -> (sum=w754:dbl)
                    n146 = Divide(x=w754, y=1000.0) -> (x/y=w753:dbl)
                    n147 = call <vilib>:"Peak Detector.vi"("peaks/valleys"=enum32{"Peaks", "Valleys"}."Peaks", "threshold"=w753, "X"=w752) -> ("Amplitudes"=w758:dbl[], "Locations"=→"Locations C3":dbl[])  [unwired: 4 in, 3 out]
                    n148 = Array Size(array=w758) -> (size(s)=w759:i32)
                    n149 = Greater Or Equal?(x=w759, y=1) -> (x >= y?=w757:bool)
                    "C3" <- w757
                    n150 = case shown="True" w757 {
                      tunnel: w756 -> [_ _]
                      frame False {
                      }
                      frame True {
                      }
                    }
                  }
                }
                n151 = case shown="True" w737 {
                  tunnel: w662 -> [_ w797]
                  frame False {
                  }
                  frame True {
                    n152 = To Double Precision Float(number=w797) -> (double precision float=w796:dbl[])
                    n153 = Add Array Elements(numeric array=w796) -> (sum=w795:dbl)
                    n154 = Divide(x=w795, y=1000.0) -> (x/y=w793:dbl)
                    n155 = call <vilib>:"Peak Detector.vi"("peaks/valleys"=enum32{"Peaks", "Valleys"}."Peaks", "threshold"=w793, "X"=w796) -> ("Amplitudes"=w799:dbl[], "Locations"=w792:dbl[])  [unwired: 4 in, 3 out]
                    "Locations C0" <- w792
                    n156 = Array Max & Min(array=w792) -> (max value=→"C0 max value":dbl, max index (indices)=→"C0 index position":i32)  [unwired: 2 out]
                    n157 = Array Size(array=w799) -> (size(s)=w800:i32)
                    n158 = Greater Or Equal?(x=w800, y=1) -> (x >= y?=w798:bool)
                    "C0" <- w798
                    n159 = case shown="True" w798 {
                      tunnel: w797 -> [_ w803]
                      frame False {
                      }
                      frame True {
                        "Channel 32" <- w803
                      }
                    }
                  }
                }
                n160 = case shown="True" w716 {
                  tunnel: w712 -> [_ w769]
                  frame False {
                  }
                  frame True {
                    n161 = To Double Precision Float(number=w769) -> (double precision float=w765:dbl[])
                    n162 = Add Array Elements(numeric array=w765) -> (sum=w768:dbl)
                    n163 = Divide(x=w768, y=1000.0) -> (x/y=w766:dbl)
                    n164 = call <vilib>:"Peak Detector.vi"("peaks/valleys"=enum32{"Peaks", "Valleys"}."Peaks", "threshold"=w766, "X"=w765) -> ("Amplitudes"=w771:dbl[], "Locations"=→"Locations C2":dbl[])  [unwired: 4 in, 3 out]
                    n165 = Array Size(array=w771) -> (size(s)=w772:i32)
                    n166 = Greater Or Equal?(x=w772, y=1) -> (x >= y?=w770:bool)
                    "C2" <- w770
                    n167 = case shown="True" w770 {
                      frame False {
                      }
                      frame True {
                      }
                    }
                  }
                }
                n168 = case shown="True" w735 {
                  tunnel: w725 -> [_ w782]
                  frame False {
                  }
                  frame True {
                    n169 = To Double Precision Float(number=w782) -> (double precision float=w779:dbl[])
                    n170 = Add Array Elements(numeric array=w779) -> (sum=w780:dbl)
                    n171 = Divide(x=w780, y=1000.0) -> (x/y=w778:dbl)
                    n172 = call <vilib>:"Peak Detector.vi"("peaks/valleys"=enum32{"Peaks", "Valleys"}."Peaks", "threshold"=w778, "X"=w779) -> ("Amplitudes"=w784:dbl[], "Locations"=→"Locations C1":dbl[])  [unwired: 4 in, 3 out]
                    n173 = Array Size(array=w784) -> (size(s)=w785:i32)
                    n174 = Greater Or Equal?(x=w785, y=1) -> (x >= y?=w783:bool)
                    "C1" <- w783
                    n175 = case shown="True" w783 {
                      tunnel: w782 -> [_ _]
                      frame False {
                      }
                      frame True {
                      }
                    }
                  }
                }
                "Ring 0" <- TRUE ("Ring 0")
              }
              frame 4 {
                # "C7"
                # "C6"
                # "C5"
                # "C4"
                n176 = VISA Read(VISA resource name=w897, byte count=u32 8, error in (no error)=w896) -> (read buffer=w895:string)  [unwired: 3 out]
                n177 = String To Byte Array(string=w895) -> (unsigned byte array=w848:u8[])
                n178 = Index Array(array=w848, index=1) -> (element=w882:u8)
                n179 = Index Array(array=w848, index=0) -> (element=w884:u8)
                n180 = Index Array(array=w848, index=3) -> (element=w879:u8)
                n181 = Index Array(array=w848, index=5) -> (element=w861:u8)
                n182 = Index Array(array=w848, index=2) -> (element=w877:u8)
                n183 = Index Array(array=w848, index=4) -> (element=w863:u8)
                n184 = Index Array(array=w848, index=7) -> (element=w854:u8)
                n185 = Index Array(array=w848, index=6) -> (element=w852:u8)
                n186 = Join Numbers(hi=w882, lo=w884) -> ((hi.lo)=w886:u16)
                n187 = Join Numbers(hi=w879, lo=w877) -> ((hi.lo)=w875:u16)
                n188 = Join Numbers(hi=w861, lo=w863) -> ((hi.lo)=w865:u16)
                n189 = Join Numbers(hi=w854, lo=w852) -> ((hi.lo)=w850:u16)
                n190 = To Word Integer(number=w886) -> (16bit integer=w806:i16)
                "Channel 4" <- w806
                n191 = property on="C4" class="DigNum (strict)"() -> ("Value"=w881:u16)  [unwired: 2 in, 2 out]
                n192 = To Word Integer(number=w875) -> (16bit integer=w880:i16)
                n193 = To Word Integer(number=w865) -> (16bit integer=w860:i16)
                n194 = To Word Integer(number=w850) -> (16bit integer=w849:i16)
                n195 = property on="C5" class="DigNum (strict)"() -> ("Value"=w870:u16)  [unwired: 2 in, 2 out]
                n196 = property on="C7" class="DigNum (strict)"() -> ("Value"=w839:u16)  [unwired: 2 in, 2 out]
                n197 = property on="C6" class="DigNum (strict)"() -> ("Value"=w859:u16)  [unwired: 2 in, 2 out]
                n198 = Add(x=u16 1, y=w881) -> (x+y=w888:u16)
                n199 = Equal?(x=w888, y=u16 1000) -> (x = y?=w890:bool)
                n200 = Add(x=u16 1, y=w839) -> (x+y=w857:u16)
                n201 = Equal?(x=w857, y=u16 1000) -> (x = y?=w855:bool)
                n202 = Add(x=u16 1, y=w870) -> (x+y=w873:u16)
                n203 = Equal?(x=w873, y=u16 1000) -> (x = y?=w871:bool)
                n204 = Add(x=u16 1, y=w859) -> (x+y=w867:u16)
                n205 = Equal?(x=w867, y=u16 1000) -> (x = y?=w869:bool)
                n206 = local write "Ring 0"(FALSE ("Ring 0")) -> ()
                n207 = local write "Ring 3"(FALSE ("Ring 0")) -> ()
                n208 = case shown="1000" w888 {
                  selector: w888 -> [w955 _]
                  frame 0, Default {
                    n209 = property on="C4" class="DigNum (strict)"("Value"=w955) -> ()  [unwired: 2 in, 2 out]
                  }
                  frame 1000 {
                    n210 = property on="C4" class="DigNum (strict)"("Value"=0) -> ()  [unwired: 2 in, 2 out]
                  }
                }
                n211 = case shown="1000" w857 {
                  selector: w857 -> [w911 _]
                  frame 0, Default {
                    n212 = property on="C7" class="DigNum (strict)"("Value"=w911) -> ()  [unwired: 2 in, 2 out]
                  }
                  frame 1000 {
                    n213 = property on="C7" class="DigNum (strict)"("Value"=0) -> ()  [unwired: 2 in, 2 out]
                  }
                }
                n214 = case shown="1000" w873 {
                  selector: w873 -> [w939 _]
                  frame 0, Default {
                    n215 = property on="C5" class="DigNum (strict)"("Value"=w939) -> ()  [unwired: 2 in, 2 out]
                  }
                  frame 1000 {
                    n216 = property on="C5" class="DigNum (strict)"("Value"=0) -> ()  [unwired: 2 in, 2 out]
                  }
                }
                n217 = case shown="1000" w867 {
                  selector: w867 -> [w925 _]
                  frame 0, Default {
                    n218 = property on="C6" class="DigNum (strict)"("Value"=w925) -> ()  [unwired: 2 in, 2 out]
                  }
                  frame 1000 {
                    n219 = property on="C6" class="DigNum (strict)"("Value"=0) -> ()  [unwired: 2 in, 2 out]
                  }
                }
                n220 = local write "Ring 7"(FALSE ("Ring 0")) -> ()
                n221 = local write "Ring 4"(FALSE ("Ring 0")) -> ()
                n222 = local write "Ring 6"(FALSE ("Ring 0")) -> ()
                n223 = local write "Ring 5"(FALSE ("Ring 0")) -> ()
                n224 = local write "Ring 2"(FALSE ("Ring 0")) -> ()
                n225 = Replace Array Subset(array=w844, new element=w849, index=w839) -> (w840:i16[])
                n226 = Replace Array Subset(array=w846, new element=w880, index=w870) -> (w842:i16[])
                n227 = Replace Array Subset(array=w845, new element=w860, index=w859) -> (w841:i16[])
                n228 = Replace Array Subset(array=w847, new element=w806, index=w881) -> (w843:i16[])
                n229 = case shown="True" w890 {
                  tunnel: w843 -> [_ w948]
                  frame False {
                  }
                  frame True {
                    n230 = To Double Precision Float(number=w948) -> (double precision float=w944:dbl[])
                    n231 = Add Array Elements(numeric array=w944) -> (sum=w947:dbl)
                    n232 = Divide(x=w947, y=1000.0) -> (x/y=w945:dbl)
                    n233 = call <vilib>:"Peak Detector.vi"("peaks/valleys"=enum32{"Peaks", "Valleys"}."Peaks", "threshold"=w945, "X"=w944) -> ("Amplitudes"=w950:dbl[], "Locations"=w942:dbl[])  [unwired: 4 in, 3 out]
                    "Locations C4" <- w942
                    n234 = Array Max & Min(array=w942) -> (max value=→"C4  max value":dbl, max index (indices)=→"Ch4 index position":i32)  [unwired: 2 out]
                    n235 = Array Size(array=w950) -> (size(s)=w951:i32)
                    n236 = Greater Or Equal?(x=w951, y=1) -> (x >= y?=w949:bool)
                    "C4" <- w949
                    n237 = case shown="True" w949 {
                      tunnel: w948 -> [_ w954]
                      frame False {
                      }
                      frame True {
                        "Channel 33" <- w954
                      }
                    }
                  }
                }
                n238 = case shown="True" w855 {
                  tunnel: w840 -> [_ w904]
                  frame False {
                  }
                  frame True {
                    n239 = To Double Precision Float(number=w904) -> (double precision float=w900:dbl[])
                    n240 = Add Array Elements(numeric array=w900) -> (sum=w902:dbl)
                    n241 = Divide(x=w902, y=1000.0) -> (x/y=w901:dbl)
                    n242 = call <vilib>:"Peak Detector.vi"("peaks/valleys"=enum32{"Peaks", "Valleys"}."Peaks", "threshold"=w901, "X"=w900) -> ("Amplitudes"=w906:dbl[], "Locations"=→"Locations C7":dbl[])  [unwired: 4 in, 3 out]
                    n243 = Array Size(array=w906) -> (size(s)=w907:i32)
                    n244 = Greater Or Equal?(x=w907, y=1) -> (x >= y?=w905:bool)
                    "C7" <- w905
                    n245 = case shown="True" w905 {
                      tunnel: w904 -> [_ w910]
                      frame False {
                      }
                      frame True {
                        "Channel 7" <- w910
                      }
                    }
                  }
                }
                n246 = case shown="True" w871 {
                  tunnel: w842 -> [_ w932]
                  frame False {
                  }
                  frame True {
                    n247 = To Double Precision Float(number=w932) -> (double precision float=w929:dbl[])
                    n248 = Add Array Elements(numeric array=w929) -> (sum=w930:dbl)
                    n249 = Divide(x=w930, y=1000.0) -> (x/y=w928:dbl)
                    n250 = call <vilib>:"Peak Detector.vi"("peaks/valleys"=enum32{"Peaks", "Valleys"}."Peaks", "threshold"=w928, "X"=w929) -> ("Amplitudes"=w934:dbl[], "Locations"=→"Locations C5":dbl[])  [unwired: 4 in, 3 out]
                    n251 = Array Size(array=w934) -> (size(s)=w935:i32)
                    n252 = Greater Or Equal?(x=w935, y=1) -> (x >= y?=w933:bool)
                    "C5" <- w933
                    n253 = case shown="True" w933 {
                      tunnel: w932 -> [_ w938]
                      frame False {
                      }
                      frame True {
                        "Channel 5" <- w938
                      }
                    }
                  }
                }
                n254 = case shown="True" w869 {
                  tunnel: w841 -> [_ w918]
                  frame False {
                  }
                  frame True {
                    n255 = To Double Precision Float(number=w918) -> (double precision float=w914:dbl[])
                    n256 = Add Array Elements(numeric array=w914) -> (sum=w917:dbl)
                    n257 = Divide(x=w917, y=1000.0) -> (x/y=w915:dbl)
                    n258 = call <vilib>:"Peak Detector.vi"("peaks/valleys"=enum32{"Peaks", "Valleys"}."Peaks", "threshold"=w915, "X"=w914) -> ("Amplitudes"=w920:dbl[], "Locations"=→"Locations C6":dbl[])  [unwired: 4 in, 3 out]
                    n259 = Array Size(array=w920) -> (size(s)=w921:i32)
                    n260 = Greater Or Equal?(x=w921, y=1) -> (x >= y?=w919:bool)
                    "C6" <- w919
                    n261 = case shown="True" w919 {
                      tunnel: w918 -> [_ w924]
                      frame False {
                      }
                      frame True {
                        "Channel 6" <- w924
                      }
                    }
                  }
                }
                "Ring 1" <- TRUE ("Ring 1")
              }
              frame 8 {
                # "C11"
                # "C10"
                # "C9"
                # "C8"
                n262 = VISA Read(VISA resource name=w1048, byte count=u32 8, error in (no error)=w1047) -> (read buffer=w1046:string)  [unwired: 3 out]
                n263 = String To Byte Array(string=w1046) -> (unsigned byte array=w993:u8[])
                n264 = Index Array(array=w993, index=1) -> (element=w1031:u8)
                n265 = Index Array(array=w993, index=0) -> (element=w1029:u8)
                n266 = Index Array(array=w993, index=5) -> (element=w1009:u8)
                n267 = Index Array(array=w993, index=3) -> (element=w1023:u8)
                n268 = Index Array(array=w993, index=4) -> (element=w1007:u8)
                n269 = Index Array(array=w993, index=2) -> (element=w1025:u8)
                n270 = Index Array(array=w993, index=5) -> (element=w996:u8)
                n271 = Index Array(array=w993, index=4) -> (element=w998:u8)
                n272 = Join Numbers(hi=w1031, lo=w1029) -> ((hi.lo)=w1032:u16)
                n273 = Join Numbers(hi=w1009, lo=w1007) -> ((hi.lo)=w1010:u16)
                n274 = Join Numbers(hi=w1023, lo=w1025) -> ((hi.lo)=w1022:u16)
                n275 = Join Numbers(hi=w996, lo=w998) -> ((hi.lo)=w995:u16)
                n276 = property on="C9" class="DigNum (strict)"() -> ("Value"=w1016:u16)  [unwired: 2 in, 2 out]
                n277 = property on="C10" class="DigNum (strict)"() -> ("Value"=w1005:u16)  [unwired: 2 in, 2 out]
                n278 = property on="C8" class="DigNum (strict)"() -> ("Value"=w1027:u16)  [unwired: 2 in, 2 out]
                n279 = property on="C11" class="DigNum (strict)"() -> ("Value"=w994:u16)  [unwired: 2 in, 2 out]
                n280 = local write "Ring 0"(FALSE ("Ring 0")) -> ()
                n281 = local write "Ring 3"(FALSE ("Ring 0")) -> ()
                n282 = local write "Ring 7"(FALSE ("Ring 0")) -> ()
                n283 = Add(x=u16 1, y=w1027) -> (x+y=w1035:u16)
                n284 = Equal?(x=w1035, y=u16 1000) -> (x = y?=w1037:bool)
                n285 = Add(x=u16 1, y=w1005) -> (x+y=w1013:u16)
                n286 = Equal?(x=w1013, y=u16 1000) -> (x = y?=w1015:bool)
                n287 = Add(x=u16 1, y=w1016) -> (x+y=w1019:u16)
                n288 = Equal?(x=w1019, y=u16 1000) -> (x = y?=w1017:bool)
                n289 = Add(x=u16 1, y=w994) -> (x+y=w1002:u16)
                n290 = Equal?(x=w1002, y=u16 1000) -> (x = y?=w1000:bool)
                n291 = To Word Integer(number=w1032) -> (16bit integer=w1033:i16)
                n292 = To Word Integer(number=w1010) -> (16bit integer=w1011:i16)
                n293 = To Word Integer(number=w1022) -> (16bit integer=w1021:i16)
                n294 = To Word Integer(number=w995) -> (16bit integer=w1004:i16)
                n295 = local write "Ring 4"(FALSE ("Ring 0")) -> ()
                n296 = local write "Ring 1"(FALSE ("Ring 0")) -> ()
                n297 = case shown="100" w1035 {
                  selector: w1035 -> [w1105 _]
                  frame 0, Default {
                    n298 = property on="C8" class="DigNum (strict)"("Value"=w1105) -> ()  [unwired: 2 in, 2 out]
                  }
                  frame 100 {
                    n299 = property on="C8" class="DigNum (strict)"("Value"=0) -> ()  [unwired: 2 in, 2 out]
                  }
                }
                n300 = case shown="1000" w1013 {
                  selector: w1013 -> [w1076 _]
                  frame 0, Default {
                    n301 = property on="C10" class="DigNum (strict)"("Value"=w1076) -> ()  [unwired: 2 in, 2 out]
                  }
                  frame 1000 {
                    n302 = property on="C10" class="DigNum (strict)"("Value"=0) -> ()  [unwired: 2 in, 2 out]
                  }
                }
                n303 = case shown="0, Default" w1019 {
                  selector: w1019 -> [w1090 _]
                  frame 0, Default {
                    n304 = property on="C9" class="DigNum (strict)"("Value"=w1090) -> ()  [unwired: 2 in, 2 out]
                  }
                  frame 100 {
                    n305 = property on="C9" class="DigNum (strict)"("Value"=0) -> ()  [unwired: 2 in, 2 out]
                  }
                }
                n306 = case shown="1000" w1002 {
                  selector: w1002 -> [w1062 _]
                  frame 0, Default {
                    n307 = property on="C11" class="DigNum (strict)"("Value"=w1062) -> ()  [unwired: 2 in, 2 out]
                  }
                  frame 1000 {
                    n308 = property on="C11" class="DigNum (strict)"("Value"=0) -> ()  [unwired: 2 in, 2 out]
                  }
                }
                n309 = local write "Ring 6"(FALSE ("Ring 0")) -> ()
                n310 = local write "Ring 5"(FALSE ("Ring 0")) -> ()
                n311 = Replace Array Subset(array=w992, new element=w1033, index=w1027) -> (w988:i16[])
                n312 = Replace Array Subset(array=w990, new element=w1011, index=w1005) -> (w986:i16[])
                n313 = Replace Array Subset(array=w991, new element=w1021, index=w1016) -> (w987:i16[])
                n314 = Replace Array Subset(array=w989, new element=w1004, index=w994) -> (w985:i16[])
                n315 = case shown="True" w1037 {
                  tunnel: w988 -> [_ w1098]
                  frame False {
                  }
                  frame True {
                    n316 = To Double Precision Float(number=w1098) -> (double precision float=w1094:dbl[])
                    n317 = Add Array Elements(numeric array=w1094) -> (sum=w1097:dbl)
                    n318 = Divide(x=w1097, y=1000.0) -> (x/y=w1095:dbl)
                    n319 = call <vilib>:"Peak Detector.vi"("peaks/valleys"=enum32{"Peaks", "Valleys"}."Peaks", "threshold"=w1095, "X"=w1094) -> ("Amplitudes"=w1100:dbl[], "Locations"=w1093:dbl[])  [unwired: 4 in, 3 out]
                    "Locations C8" <- w1093
                    n320 = Array Size(array=w1100) -> (size(s)=w1101:i32)
                    n321 = Greater Or Equal?(x=w1101, y=1) -> (x >= y?=w1099:bool)
                    "C8" <- w1099
                    n322 = case shown="True" w1099 {
                      tunnel: w1098 -> [_ w1104]
                      frame False {
                      }
                      frame True {
                        "Channel 8" <- w1104
                      }
                    }
                    n323 = Array Max & Min(array=w1093) -> (max index (indices)=→"Channel 8 max":i32)  [unwired: 3 out]
                  }
                }
                n324 = case shown="True" w1015 {
                  tunnel: w986 -> [_ w1069]
                  frame False {
                  }
                  frame True {
                    n325 = To Double Precision Float(number=w1069) -> (double precision float=w1065:dbl[])
                    n326 = Add Array Elements(numeric array=w1065) -> (sum=w1068:dbl)
                    n327 = Divide(x=w1068, y=1000.0) -> (x/y=w1066:dbl)
                    n328 = call <vilib>:"Peak Detector.vi"("peaks/valleys"=enum32{"Peaks", "Valleys"}."Peaks", "threshold"=w1066, "X"=w1065) -> ("Amplitudes"=w1071:dbl[], "Locations"=→"Locations C10":dbl[])  [unwired: 4 in, 3 out]
                    n329 = Array Size(array=w1071) -> (size(s)=w1072:i32)
                    n330 = Greater Or Equal?(x=w1072, y=1) -> (x >= y?=w1070:bool)
                    "C10" <- w1070
                    n331 = case shown="True" w1070 {
                      tunnel: w1069 -> [_ w1075]
                      frame False {
                      }
                      frame True {
                        "Channel 10" <- w1075
                      }
                    }
                  }
                }
                n332 = case shown="True" w1017 {
                  tunnel: w987 -> [_ w1083]
                  frame False {
                  }
                  frame True {
                    n333 = To Double Precision Float(number=w1083) -> (double precision float=w1079:dbl[])
                    n334 = Add Array Elements(numeric array=w1079) -> (sum=w1081:dbl)
                    n335 = Divide(x=w1081, y=1000.0) -> (x/y=w1080:dbl)
                    n336 = call <vilib>:"Peak Detector.vi"("peaks/valleys"=enum32{"Peaks", "Valleys"}."Peaks", "threshold"=w1080, "X"=w1079) -> ("Amplitudes"=w1085:dbl[], "Locations"=→"Locations C9":dbl[])  [unwired: 4 in, 3 out]
                    n337 = Array Size(array=w1085) -> (size(s)=w1086:i32)
                    n338 = Greater Or Equal?(x=w1086, y=1) -> (x >= y?=w1084:bool)
                    "C9" <- w1084
                    n339 = case shown="True" w1084 {
                      tunnel: w1083 -> [_ w1089]
                      frame False {
                      }
                      frame True {
                        "Channel 9" <- w1089
                      }
                    }
                  }
                }
                n340 = case shown="True" w1000 {
                  tunnel: w985 -> [_ w1055]
                  frame False {
                  }
                  frame True {
                    n341 = To Double Precision Float(number=w1055) -> (double precision float=w1051:dbl[])
                    n342 = Add Array Elements(numeric array=w1051) -> (sum=w1053:dbl)
                    n343 = Divide(x=w1053, y=1000.0) -> (x/y=w1052:dbl)
                    n344 = call <vilib>:"Peak Detector.vi"("peaks/valleys"=enum32{"Peaks", "Valleys"}."Peaks", "threshold"=w1052, "X"=w1051) -> ("Amplitudes"=w1057:dbl[], "Locations"=→"Locations C11":dbl[])  [unwired: 4 in, 3 out]
                    n345 = Array Size(array=w1057) -> (size(s)=w1058:i32)
                    n346 = Greater Or Equal?(x=w1058, y=1) -> (x >= y?=w1056:bool)
                    "C11" <- w1056
                    n347 = case shown="True" w1056 {
                      tunnel: w1055 -> [_ w1061]
                      frame False {
                      }
                      frame True {
                        "Channel 11" <- w1061
                      }
                    }
                  }
                }
                "Ring 2" <- TRUE ("Ring 2")
              }
              frame 12 {
                # "C15"
                # "C14"
                # "C13"
                # "C12"
                n348 = VISA Read(VISA resource name=w1198, byte count=u32 8, error in (no error)=w1197) -> (read buffer=w1196:string)  [unwired: 3 out]
                n349 = String To Byte Array(string=w1196) -> (unsigned byte array=w1143:u8[])
                n350 = Index Array(array=w1143, index=7) -> (element=w1150:u8)
                n351 = Index Array(array=w1143, index=5) -> (element=w1157:u8)
                n352 = Index Array(array=w1143, index=6) -> (element=w1152:u8)
                n353 = Index Array(array=w1143, index=4) -> (element=w1155:u8)
                n354 = Index Array(array=w1143, index=3) -> (element=w1170:u8)
                n355 = Index Array(array=w1143, index=2) -> (element=w1172:u8)
                n356 = Index Array(array=w1143, index=1) -> (element=w1177:u8)
                n357 = Index Array(array=w1143, index=0) -> (element=w1175:u8)
                n358 = property on="C15" class="DigNum (strict)"() -> ("Value"=w1140:u16)  [unwired: 2 in, 2 out]
                n359 = Join Numbers(hi=w1150, lo=w1152) -> ((hi.lo)=w1149:u16)
                n360 = Join Numbers(hi=w1157, lo=w1155) -> ((hi.lo)=w1158:u16)
                n361 = Join Numbers(hi=w1170, lo=w1172) -> ((hi.lo)=w1169:u16)
                n362 = Join Numbers(hi=w1177, lo=w1175) -> ((hi.lo)=w1178:u16)
                n363 = property on="C14" class="DigNum (strict)"() -> ("Value"=w1139:u16)  [unwired: 2 in, 2 out]
                n364 = property on="C12" class="DigNum (strict)"() -> ("Value"=w1142:u16)  [unwired: 2 in, 2 out]
                n365 = property on="C13" class="DigNum (strict)"() -> ("Value"=w1141:u16)  [unwired: 2 in, 2 out]
                n366 = Add(x=u16 1, y=w1140) -> (x+y=w1146:u16)
                n367 = Equal?(x=w1146, y=u16 1000) -> (x = y?=w1144:bool)
                n368 = Add(x=u16 1, y=w1139) -> (x+y=w1161:u16)
                n369 = Equal?(x=w1161, y=u16 1000) -> (x = y?=w1163:bool)
                n370 = Add(x=u16 1, y=w1141) -> (x+y=w1166:u16)
                n371 = Equal?(x=w1166, y=u16 1000) -> (x = y?=w1164:bool)
                n372 = Add(x=u16 1, y=w1142) -> (x+y=w1181:u16)
                n373 = Equal?(x=w1181, y=u16 1000) -> (x = y?=w1183:bool)
                n374 = To Word Integer(number=w1149) -> (16bit integer=w1148:i16)
                n375 = To Word Integer(number=w1158) -> (16bit integer=w1159:i16)
                n376 = To Word Integer(number=w1169) -> (16bit integer=w1168:i16)
                n377 = local write "Ring 0"(FALSE ("Ring 0")) -> ()
                n378 = To Word Integer(number=w1178) -> (16bit integer=w1179:i16)
                n379 = case shown="1000" w1146 {
                  selector: w1146 -> [w1212 _]
                  frame 0, Default {
                    n380 = property on="C15" class="DigNum (strict)"("Value"=w1212) -> ()  [unwired: 2 in, 2 out]
                  }
                  frame 1000 {
                    n381 = property on="C15" class="DigNum (strict)"("Value"=0) -> ()  [unwired: 2 in, 2 out]
                  }
                }
                n382 = case shown="1000" w1161 {
                  selector: w1161 -> [w1226 _]
                  frame 0, Default {
                    n383 = property on="C14" class="DigNum (strict)"("Value"=w1226) -> ()  [unwired: 2 in, 2 out]
                  }
                  frame 1000 {
                    n384 = property on="C14" class="DigNum (strict)"("Value"=0) -> ()  [unwired: 2 in, 2 out]
                  }
                }
                n385 = local write "Ring 7"(FALSE ("Ring 0")) -> ()
                n386 = case shown="1000" w1166 {
                  selector: w1166 -> [w1240 _]
                  frame 0, Default {
                    n387 = property on="C13" class="DigNum (strict)"("Value"=w1240) -> ()  [unwired: 2 in, 2 out]
                  }
                  frame 1000 {
                    n388 = property on="C13" class="DigNum (strict)"("Value"=0) -> ()  [unwired: 2 in, 2 out]
                  }
                }
                n389 = case shown="1000" w1181 {
                  selector: w1181 -> [w1254 _]
                  frame 0, Default {
                    n390 = property on="C12" class="DigNum (strict)"("Value"=w1254) -> ()  [unwired: 2 in, 2 out]
                  }
                  frame 1000 {
                    n391 = property on="C12" class="DigNum (strict)"("Value"=0) -> ()  [unwired: 2 in, 2 out]
                  }
                }
                n392 = local write "Ring 4"(FALSE ("Ring 0")) -> ()
                n393 = local write "Ring 1"(FALSE ("Ring 0")) -> ()
                n394 = local write "Ring 6"(FALSE ("Ring 0")) -> ()
                n395 = local write "Ring 5"(FALSE ("Ring 0")) -> ()
                n396 = local write "Ring 2"(FALSE ("Ring 0")) -> ()
                n397 = Replace Array Subset(array=w1138, new element=w1148, index=w1140) -> (w1131:i16[])
                n398 = Replace Array Subset(array=w1137, new element=w1159, index=w1139) -> (w1132:i16[])
                n399 = Replace Array Subset(array=w1136, new element=w1168, index=w1141) -> (w1133:i16[])
                n400 = Replace Array Subset(array=w1135, new element=w1179, index=w1142) -> (w1134:i16[])
                n401 = case shown="True" w1163 {
                  tunnel: w1132 -> [_ w1219]
                  frame False {
                  }
                  frame True {
                    n402 = To Double Precision Float(number=w1219) -> (double precision float=w1215:dbl[])
                    n403 = Add Array Elements(numeric array=w1215) -> (sum=w1218:dbl)
                    n404 = Divide(x=w1218, y=1000.0) -> (x/y=w1216:dbl)
                    n405 = call <vilib>:"Peak Detector.vi"("peaks/valleys"=enum32{"Peaks", "Valleys"}."Peaks", "threshold"=w1216, "X"=w1215) -> ("Amplitudes"=w1221:dbl[], "Locations"=→"Locations C14":dbl[])  [unwired: 4 in, 3 out]
                    n406 = Array Size(array=w1221) -> (size(s)=w1222:i32)
                    n407 = Greater Or Equal?(x=w1222, y=1) -> (x >= y?=w1220:bool)
                    "C14" <- w1220
                    n408 = case shown="True" w1220 {
                      tunnel: w1219 -> [_ w1225]
                      frame False {
                      }
                      frame True {
                        "Channel 14" <- w1225
                      }
                    }
                  }
                }
                n409 = case shown="True" w1144 {
                  tunnel: w1131 -> [_ w1205]
                  frame False {
                  }
                  frame True {
                    n410 = To Double Precision Float(number=w1205) -> (double precision float=w1201:dbl[])
                    n411 = Add Array Elements(numeric array=w1201) -> (sum=w1203:dbl)
                    n412 = Divide(x=w1203, y=1000.0) -> (x/y=w1202:dbl)
                    n413 = call <vilib>:"Peak Detector.vi"("peaks/valleys"=enum32{"Peaks", "Valleys"}."Peaks", "threshold"=w1202, "X"=w1201) -> ("Amplitudes"=w1207:dbl[], "Locations"=→"Locations C15":dbl[])  [unwired: 4 in, 3 out]
                    n414 = Array Size(array=w1207) -> (size(s)=w1208:i32)
                    n415 = Greater Or Equal?(x=w1208, y=1) -> (x >= y?=w1206:bool)
                    "C15" <- w1206
                    n416 = case shown="True" w1206 {
                      tunnel: w1205 -> [_ w1211]
                      frame False {
                      }
                      frame True {
                        "Channel 15" <- w1211
                      }
                    }
                  }
                }
                n417 = case shown="True" w1164 {
                  tunnel: w1133 -> [_ w1233]
                  frame False {
                  }
                  frame True {
                    n418 = To Double Precision Float(number=w1233) -> (double precision float=w1230:dbl[])
                    n419 = Add Array Elements(numeric array=w1230) -> (sum=w1231:dbl)
                    n420 = Divide(x=w1231, y=1000.0) -> (x/y=w1229:dbl)
                    n421 = call <vilib>:"Peak Detector.vi"("peaks/valleys"=enum32{"Peaks", "Valleys"}."Peaks", "threshold"=w1229, "X"=w1230) -> ("Amplitudes"=w1235:dbl[], "Locations"=→"Locations 13":dbl[])  [unwired: 4 in, 3 out]
                    n422 = Array Size(array=w1235) -> (size(s)=w1236:i32)
                    n423 = Greater Or Equal?(x=w1236, y=1) -> (x >= y?=w1234:bool)
                    "C13" <- w1234
                    n424 = case shown="True" w1234 {
                      tunnel: w1233 -> [_ w1239]
                      frame False {
                      }
                      frame True {
                        "Channel 13" <- w1239
                      }
                    }
                  }
                }
                n425 = case shown="True" w1183 {
                  tunnel: w1134 -> [_ w1247]
                  frame False {
                  }
                  frame True {
                    n426 = To Double Precision Float(number=w1247) -> (double precision float=w1243:dbl[])
                    n427 = Add Array Elements(numeric array=w1243) -> (sum=w1246:dbl)
                    n428 = Divide(x=w1246, y=1000.0) -> (x/y=w1244:dbl)
                    n429 = call <vilib>:"Peak Detector.vi"("peaks/valleys"=enum32{"Peaks", "Valleys"}."Peaks", "threshold"=w1244, "X"=w1243) -> ("Amplitudes"=w1249:dbl[], "Locations"=→"Locations 12":dbl[])  [unwired: 4 in, 3 out]
                    n430 = Array Size(array=w1249) -> (size(s)=w1250:i32)
                    n431 = Greater Or Equal?(x=w1250, y=1) -> (x >= y?=w1248:bool)
                    "C12" <- w1248
                    n432 = case shown="True" w1248 {
                      tunnel: w1247 -> [_ w1253]
                      frame False {
                      }
                      frame True {
                        "Channel 12" <- w1253
                      }
                    }
                  }
                }
                "Ring 3" <- TRUE ("Ring 3")
              }
              frame 16 {
                # "C19"
                # "C18"
                # "C17"
                # "C16"
                n433 = VISA Read(VISA resource name=w1347, byte count=u32 8, error in (no error)=w1346) -> (read buffer=w1345:string)  [unwired: 3 out]
                n434 = String To Byte Array(string=w1345) -> (unsigned byte array=w1284:u8[])
                n435 = Index Array(array=w1284, index=7) -> (element=w1294:u8)
                n436 = Index Array(array=w1284, index=6) -> (element=w1296:u8)
                n437 = Index Array(array=w1284, index=3) -> (element=w1314:u8)
                n438 = Index Array(array=w1284, index=5) -> (element=w1301:u8)
                n439 = Index Array(array=w1284, index=2) -> (element=w1316:u8)
                n440 = Index Array(array=w1284, index=1) -> (element=w1322:u8)
                n441 = Index Array(array=w1284, index=4) -> (element=w1299:u8)
                n442 = Index Array(array=w1284, index=0) -> (element=w1320:u8)
                n443 = Join Numbers(hi=w1294, lo=w1296) -> ((hi.lo)=w1293:u16)
                n444 = Join Numbers(hi=w1314, lo=w1316) -> ((hi.lo)=w1313:u16)
                n445 = Join Numbers(hi=w1301, lo=w1299) -> ((hi.lo)=w1302:u16)
                n446 = Join Numbers(hi=w1322, lo=w1320) -> ((hi.lo)=w1323:u16)
                n447 = property on="C19" class="DigNum (strict)"() -> ("Value"=w1287:u16)  [unwired: 2 in, 2 out]
                n448 = property on="C17" class="DigNum (strict)"() -> ("Value"=w1285:u16)  [unwired: 2 in, 2 out]
                n449 = property on="C16" class="DigNum (strict)"() -> ("Value"=w1318:u16)  [unwired: 2 in, 2 out]
                n450 = property on="C18" class="DigNum (strict)"() -> ("Value"=w1286:u16)  [unwired: 2 in, 2 out]
                n451 = Add(x=u16 1, y=w1287) -> (x+y=w1290:u16)
                n452 = Equal?(x=w1290, y=u16 1000) -> (x = y?=w1288:bool)
                n453 = Add(x=u16 1, y=w1285) -> (x+y=w1310:u16)
                n454 = Equal?(x=w1310, y=u16 1000) -> (x = y?=w1308:bool)
                n455 = Add(x=u16 1, y=w1286) -> (x+y=w1305:u16)
                n456 = Equal?(x=w1305, y=u16 1000) -> (x = y?=w1307:bool)
                n457 = Add(x=u16 1, y=w1318) -> (x+y=w1326:u16)
                n458 = Equal?(x=w1326, y=u16 1000) -> (x = y?=w1328:bool)
                n459 = To Word Integer(number=w1293) -> (16bit integer=w1292:i16)
                n460 = To Word Integer(number=w1313) -> (16bit integer=w1312:i16)
                n461 = To Word Integer(number=w1302) -> (16bit integer=w1303:i16)
                n462 = To Word Integer(number=w1323) -> (16bit integer=w1324:i16)
                n463 = case shown="1000" w1290 {
                  selector: w1290 -> [w1361 _]
                  frame 0, Default {
                    n464 = property on="C19" class="DigNum (strict)"("Value"=w1361) -> ()  [unwired: 2 in, 2 out]
                  }
                  frame 1000 {
                    n465 = property on="C19" class="DigNum (strict)"("Value"=0) -> ()  [unwired: 2 in, 2 out]
                  }
                }
                n466 = case shown="1000" w1310 {
                  selector: w1310 -> [w1389 _]
                  frame 0, Default {
                    n467 = property on="C17" class="DigNum (strict)"("Value"=w1389) -> ()  [unwired: 2 in, 2 out]
                  }
                  frame 1000 {
                    n468 = property on="C17" class="DigNum (strict)"("Value"=0) -> ()  [unwired: 2 in, 2 out]
                  }
                }
                n469 = case shown="1000" w1305 {
                  selector: w1305 -> [w1375 _]
                  frame 0, Default {
                    n470 = property on="C18" class="DigNum (strict)"("Value"=w1375) -> ()  [unwired: 2 in, 2 out]
                  }
                  frame 1000 {
                    n471 = property on="C18" class="DigNum (strict)"("Value"=0) -> ()  [unwired: 2 in, 2 out]
                  }
                }
                n472 = case shown="1000" w1326 {
                  selector: w1326 -> [w1403 _]
                  frame 0, Default {
                    n473 = property on="C16" class="DigNum (strict)"("Value"=w1403) -> ()  [unwired: 2 in, 2 out]
                  }
                  frame 1000 {
                    n474 = property on="C16" class="DigNum (strict)"("Value"=0) -> ()  [unwired: 2 in, 2 out]
                  }
                }
                n475 = local write "Ring 0"(FALSE ("Ring 0")) -> ()
                n476 = local write "Ring 3"(FALSE ("Ring 0")) -> ()
                n477 = local write "Ring 7"(FALSE ("Ring 0")) -> ()
                n478 = local write "Ring 1"(FALSE ("Ring 0")) -> ()
                n479 = local write "Ring 6"(FALSE ("Ring 0")) -> ()
                n480 = local write "Ring 5"(FALSE ("Ring 0")) -> ()
                n481 = local write "Ring 2"(FALSE ("Ring 0")) -> ()
                n482 = Replace Array Subset(array=w1276, new element=w1292, index=w1287) -> (w1280:i16[])
                n483 = Replace Array Subset(array=w1278, new element=w1312, index=w1285) -> (w1282:i16[])
                n484 = Replace Array Subset(array=w1277, new element=w1303, index=w1286) -> (w1281:i16[])
                n485 = Replace Array Subset(array=w1279, new element=w1324, index=w1318) -> (w1283:i16[])
                n486 = case shown="True" w1328 {
                  tunnel: w1283 -> [_ w1396]
                  frame False {
                  }
                  frame True {
                    n487 = To Double Precision Float(number=w1396) -> (double precision float=w1392:dbl[])
                    n488 = Add Array Elements(numeric array=w1392) -> (sum=w1395:dbl)
                    n489 = Divide(x=w1395, y=1000.0) -> (x/y=w1393:dbl)
                    n490 = call <vilib>:"Peak Detector.vi"("peaks/valleys"=enum32{"Peaks", "Valleys"}."Peaks", "threshold"=w1393, "X"=w1392) -> ("Amplitudes"=w1398:dbl[], "Locations"=→"Locations C16":dbl[])  [unwired: 4 in, 3 out]
                    n491 = Array Size(array=w1398) -> (size(s)=w1399:i32)
                    n492 = Greater Or Equal?(x=w1399, y=1) -> (x >= y?=w1397:bool)
                    "C16" <- w1397
                    n493 = case shown="True" w1397 {
                      tunnel: w1396 -> [_ w1402]
                      frame False {
                      }
                      frame True {
                        "Channel 16" <- w1402
                      }
                    }
                  }
                }
                n494 = case shown="True" w1288 {
                  tunnel: w1280 -> [_ w1354]
                  frame False {
                  }
                  frame True {
                    n495 = To Double Precision Float(number=w1354) -> (double precision float=w1350:dbl[])
                    n496 = Add Array Elements(numeric array=w1350) -> (sum=w1352:dbl)
                    n497 = Divide(x=w1352, y=1000.0) -> (x/y=w1351:dbl)
                    n498 = call <vilib>:"Peak Detector.vi"("peaks/valleys"=enum32{"Peaks", "Valleys"}."Peaks", "threshold"=w1351, "X"=w1350) -> ("Amplitudes"=w1356:dbl[], "Locations"=→"Locations C19":dbl[])  [unwired: 4 in, 3 out]
                    n499 = Array Size(array=w1356) -> (size(s)=w1357:i32)
                    n500 = Greater Or Equal?(x=w1357, y=1) -> (x >= y?=w1355:bool)
                    "C19" <- w1355
                    n501 = case shown="True" w1355 {
                      tunnel: w1354 -> [_ w1360]
                      frame False {
                      }
                      frame True {
                        "Channel 19" <- w1360
                      }
                    }
                  }
                }
                n502 = case shown="True" w1308 {
                  tunnel: w1282 -> [_ w1382]
                  frame False {
                  }
                  frame True {
                    n503 = To Double Precision Float(number=w1382) -> (double precision float=w1378:dbl[])
                    n504 = Add Array Elements(numeric array=w1378) -> (sum=w1380:dbl)
                    n505 = Divide(x=w1380, y=1000.0) -> (x/y=w1379:dbl)
                    n506 = call <vilib>:"Peak Detector.vi"("peaks/valleys"=enum32{"Peaks", "Valleys"}."Peaks", "threshold"=w1379, "X"=w1378) -> ("Amplitudes"=w1384:dbl[], "Locations"=→"Locations C17":dbl[])  [unwired: 4 in, 3 out]
                    n507 = Array Size(array=w1384) -> (size(s)=w1385:i32)
                    n508 = Greater Or Equal?(x=w1385, y=1) -> (x >= y?=w1383:bool)
                    "C17" <- w1383
                    n509 = case shown="True" w1383 {
                      tunnel: w1382 -> [_ w1388]
                      frame False {
                      }
                      frame True {
                        "Channel 17" <- w1388
                      }
                    }
                  }
                }
                n510 = case shown="True" w1307 {
                  tunnel: w1281 -> [_ w1368]
                  frame False {
                  }
                  frame True {
                    n511 = To Double Precision Float(number=w1368) -> (double precision float=w1364:dbl[])
                    n512 = Add Array Elements(numeric array=w1364) -> (sum=w1367:dbl)
                    n513 = Divide(x=w1367, y=1000.0) -> (x/y=w1365:dbl)
                    n514 = call <vilib>:"Peak Detector.vi"("peaks/valleys"=enum32{"Peaks", "Valleys"}."Peaks", "threshold"=w1365, "X"=w1364) -> ("Amplitudes"=w1370:dbl[], "Locations"=→"Locations C18":dbl[])  [unwired: 4 in, 3 out]
                    n515 = Array Size(array=w1370) -> (size(s)=w1371:i32)
                    n516 = Greater Or Equal?(x=w1371, y=1) -> (x >= y?=w1369:bool)
                    "C18" <- w1369
                    n517 = case shown="True" w1369 {
                      tunnel: w1368 -> [_ w1374]
                      frame False {
                      }
                      frame True {
                        "Channel 18" <- w1374
                      }
                    }
                  }
                }
                "Ring 4" <- TRUE ("Ring 4")
              }
              frame 20 {
                # "C23"
                # "C22"
                # "C21"
                # "C20"
                n518 = VISA Read(VISA resource name=w1496, byte count=u32 8, error in (no error)=w1495) -> (read buffer=w1494:string)  [unwired: 3 out]
                n519 = String To Byte Array(string=w1494) -> (unsigned byte array=w1431:u8[])
                n520 = Index Array(array=w1431, index=5) -> (element=w1446:u8)
                n521 = Index Array(array=w1431, index=7) -> (element=w1439:u8)
                n522 = Index Array(array=w1431, index=4) -> (element=w1444:u8)
                n523 = Index Array(array=w1431, index=6) -> (element=w1441:u8)
                n524 = Index Array(array=w1431, index=3) -> (element=w1459:u8)
                n525 = Index Array(array=w1431, index=2) -> (element=w1461:u8)
                n526 = Index Array(array=w1431, index=1) -> (element=w1467:u8)
                n527 = Index Array(array=w1431, index=0) -> (element=w1465:u8)
                n528 = Join Numbers(hi=w1446, lo=w1444) -> ((hi.lo)=w1447:u16)
                n529 = Join Numbers(hi=w1439, lo=w1441) -> ((hi.lo)=w1438:u16)
                n530 = Join Numbers(hi=w1459, lo=w1461) -> ((hi.lo)=w1458:u16)
                n531 = Join Numbers(hi=w1467, lo=w1465) -> ((hi.lo)=w1468:u16)
                n532 = local write "Ring 0"(FALSE ("Ring 0")) -> ()
                n533 = local write "Ring 3"(FALSE ("Ring 0")) -> ()
                n534 = property on="C23" class="DigNum (strict)"() -> ("Value"=w1429:u16)  [unwired: 2 in, 2 out]
                n535 = property on="C21" class="DigNum (strict)"() -> ("Value"=w1432:u16)  [unwired: 2 in, 2 out]
                n536 = property on="C22" class="DigNum (strict)"() -> ("Value"=w1430:u16)  [unwired: 2 in, 2 out]
                n537 = property on="C20" class="DigNum (strict)"() -> ("Value"=w1463:u16)  [unwired: 2 in, 2 out]
                n538 = local write "Ring 7"(FALSE ("Ring 0")) -> ()
                n539 = local write "Ring 4"(FALSE ("Ring 0")) -> ()
                n540 = local write "Ring 1"(FALSE ("Ring 0")) -> ()
                n541 = Add(x=u16 1, y=w1430) -> (x+y=w1450:u16)
                n542 = Equal?(x=w1450, y=u16 1000) -> (x = y?=w1452:bool)
                n543 = Add(x=u16 1, y=w1429) -> (x+y=w1435:u16)
                n544 = Equal?(x=w1435, y=u16 1000) -> (x = y?=w1433:bool)
                n545 = Add(x=u16 1, y=w1432) -> (x+y=w1455:u16)
                n546 = Equal?(x=w1455, y=u16 1000) -> (x = y?=w1453:bool)
                n547 = Add(x=u16 1, y=w1463) -> (x+y=w1471:u16)
                n548 = Equal?(x=w1471, y=u16 1000) -> (x = y?=w1473:bool)
                n549 = To Word Integer(number=w1447) -> (16bit integer=w1448:i16)
                n550 = local write "Ring 6"(FALSE ("Ring 0")) -> ()
                n551 = To Word Integer(number=w1438) -> (16bit integer=w1437:i16)
                n552 = To Word Integer(number=w1458) -> (16bit integer=w1457:i16)
                n553 = To Word Integer(number=w1468) -> (16bit integer=w1469:i16)
                n554 = case shown="1000" w1450 {
                  selector: w1450 -> [w1524 _]
                  frame 0, Default {
                    n555 = property on="C22" class="DigNum (strict)"("Value"=w1524) -> ()  [unwired: 2 in, 2 out]
                  }
                  frame 1000 {
                    n556 = property on="C22" class="DigNum (strict)"("Value"=0) -> ()  [unwired: 2 in, 2 out]
                  }
                }
                n557 = case shown="1000" w1435 {
                  selector: w1435 -> [w1510 _]
                  frame 0, Default {
                    n558 = property on="C23" class="DigNum (strict)"("Value"=w1510) -> ()  [unwired: 2 in, 2 out]
                  }
                  frame 1000 {
                    n559 = property on="C23" class="DigNum (strict)"("Value"=0) -> ()  [unwired: 2 in, 2 out]
                  }
                }
                n560 = case shown="1000" w1455 {
                  selector: w1455 -> [w1538 _]
                  frame 0, Default {
                    n561 = property on="C21" class="DigNum (strict)"("Value"=w1538) -> ()  [unwired: 2 in, 2 out]
                  }
                  frame 1000 {
                    n562 = property on="C21" class="DigNum (strict)"("Value"=0) -> ()  [unwired: 2 in, 2 out]
                  }
                }
                n563 = local write "Ring 2"(FALSE ("Ring 0")) -> ()
                n564 = case shown="1000" w1471 {
                  selector: w1471 -> [w1552 _]
                  frame 0, Default {
                    n565 = property on="C20" class="DigNum (strict)"("Value"=w1552) -> ()  [unwired: 2 in, 2 out]
                  }
                  frame 1000 {
                    n566 = property on="C20" class="DigNum (strict)"("Value"=0) -> ()  [unwired: 2 in, 2 out]
                  }
                }
                n567 = Replace Array Subset(array=w1422, new element=w1448, index=w1430) -> (w1426:i16[])
                n568 = Replace Array Subset(array=w1421, new element=w1437, index=w1429) -> (w1425:i16[])
                n569 = Replace Array Subset(array=w1423, new element=w1457, index=w1432) -> (w1427:i16[])
                n570 = Replace Array Subset(array=w1424, new element=w1469, index=w1463) -> (w1428:i16[])
                n571 = case shown="True" w1452 {
                  tunnel: w1426 -> [_ w1517]
                  frame False {
                  }
                  frame True {
                    n572 = To Double Precision Float(number=w1517) -> (double precision float=w1513:dbl[])
                    n573 = Add Array Elements(numeric array=w1513) -> (sum=w1516:dbl)
                    n574 = Divide(x=w1516, y=1000.0) -> (x/y=w1514:dbl)
                    n575 = call <vilib>:"Peak Detector.vi"("peaks/valleys"=enum32{"Peaks", "Valleys"}."Peaks", "threshold"=w1514, "X"=w1513) -> ("Amplitudes"=w1519:dbl[], "Locations"=→"Locations C22":dbl[])  [unwired: 4 in, 3 out]
                    n576 = Array Size(array=w1519) -> (size(s)=w1520:i32)
                    n577 = Greater Or Equal?(x=w1520, y=1) -> (x >= y?=w1518:bool)
                    "C22" <- w1518
                    n578 = case shown="True" w1518 {
                      tunnel: w1517 -> [_ w1523]
                      frame False {
                      }
                      frame True {
                        "Channel 22" <- w1523
                      }
                    }
                  }
                }
                n579 = case shown="True" w1433 {
                  tunnel: w1425 -> [_ w1503]
                  frame False {
                  }
                  frame True {
                    n580 = To Double Precision Float(number=w1503) -> (double precision float=w1500:dbl[])
                    n581 = Add Array Elements(numeric array=w1500) -> (sum=w1501:dbl)
                    n582 = Divide(x=w1501, y=1000.0) -> (x/y=w1499:dbl)
                    n583 = call <vilib>:"Peak Detector.vi"("peaks/valleys"=enum32{"Peaks", "Valleys"}."Peaks", "threshold"=w1499, "X"=w1500) -> ("Amplitudes"=w1505:dbl[], "Locations"=→"Locations C23":dbl[])  [unwired: 4 in, 3 out]
                    n584 = Array Size(array=w1505) -> (size(s)=w1506:i32)
                    n585 = Greater Or Equal?(x=w1506, y=1) -> (x >= y?=w1504:bool)
                    "C23" <- w1504
                    n586 = case shown="True" w1504 {
                      tunnel: w1503 -> [_ w1509]
                      frame False {
                      }
                      frame True {
                        "Channel 23" <- w1509
                      }
                    }
                  }
                }
                n587 = case shown="True" w1453 {
                  tunnel: w1427 -> [_ w1531]
                  frame False {
                  }
                  frame True {
                    n588 = To Double Precision Float(number=w1531) -> (double precision float=w1527:dbl[])
                    n589 = Add Array Elements(numeric array=w1527) -> (sum=w1529:dbl)
                    n590 = Divide(x=w1529, y=1000.0) -> (x/y=w1528:dbl)
                    n591 = call <vilib>:"Peak Detector.vi"("peaks/valleys"=enum32{"Peaks", "Valleys"}."Peaks", "threshold"=w1528, "X"=w1527) -> ("Amplitudes"=w1533:dbl[], "Locations"=→"Locations C21":dbl[])  [unwired: 4 in, 3 out]
                    n592 = Array Size(array=w1533) -> (size(s)=w1534:i32)
                    n593 = Greater Or Equal?(x=w1534, y=1) -> (x >= y?=w1532:bool)
                    "C21" <- w1532
                    n594 = case shown="True" w1532 {
                      tunnel: w1531 -> [_ w1537]
                      frame False {
                      }
                      frame True {
                        "Channel 21" <- w1537
                      }
                    }
                  }
                }
                n595 = case shown="True" w1473 {
                  tunnel: w1428 -> [_ w1545]
                  frame False {
                  }
                  frame True {
                    n596 = To Double Precision Float(number=w1545) -> (double precision float=w1541:dbl[])
                    n597 = Add Array Elements(numeric array=w1541) -> (sum=w1544:dbl)
                    n598 = Divide(x=w1544, y=1000.0) -> (x/y=w1542:dbl)
                    n599 = call <vilib>:"Peak Detector.vi"("peaks/valleys"=enum32{"Peaks", "Valleys"}."Peaks", "threshold"=w1542, "X"=w1541) -> ("Amplitudes"=w1547:dbl[], "Locations"=→"Locations C20":dbl[])  [unwired: 4 in, 3 out]
                    n600 = Array Size(array=w1547) -> (size(s)=w1548:i32)
                    n601 = Greater Or Equal?(x=w1548, y=1) -> (x >= y?=w1546:bool)
                    "C20" <- w1546
                    n602 = case shown="True" w1546 {
                      tunnel: w1545 -> [_ w1551]
                      frame False {
                      }
                      frame True {
                        "Channel 20" <- w1551
                      }
                    }
                  }
                }
                "Ring 5" <- TRUE ("Ring 5")
              }
              frame 24 {
                # "C27"
                # "C26"
                # "C25"
                # "C24"
                n603 = VISA Read(VISA resource name=w1645, byte count=u32 8, error in (no error)=w1644) -> (read buffer=w1643:string)  [unwired: 3 out]
                n604 = String To Byte Array(string=w1643) -> (unsigned byte array=w1574:u8[])
                n605 = Index Array(array=w1574, index=7) -> (element=w1585:u8)
                n606 = Index Array(array=w1574, index=3) -> (element=w1605:u8)
                n607 = Index Array(array=w1574, index=6) -> (element=w1587:u8)
                n608 = Index Array(array=w1574, index=5) -> (element=w1592:u8)
                n609 = Index Array(array=w1574, index=2) -> (element=w1607:u8)
                n610 = Index Array(array=w1574, index=4) -> (element=w1590:u8)
                n611 = Index Array(array=w1574, index=1) -> (element=w1624:u8)
                n612 = Index Array(array=w1574, index=0) -> (element=w1622:u8)
                n613 = Join Numbers(hi=w1585, lo=w1587) -> ((hi.lo)=w1584:u16)
                n614 = Join Numbers(hi=w1605, lo=w1607) -> ((hi.lo)=w1604:u16)
                n615 = Join Numbers(hi=w1592, lo=w1590) -> ((hi.lo)=w1593:u16)
                n616 = Join Numbers(hi=w1624, lo=w1622) -> ((hi.lo)=w1625:u16)
                n617 = property on="C26" class="DigNum (strict)"() -> ("Value"=w1577:u16)  [unwired: 2 in, 2 out]
                n618 = property on="C25" class="DigNum (strict)"() -> ("Value"=w1576:u16)  [unwired: 2 in, 2 out]
                n619 = property on="C27" class="DigNum (strict)"() -> ("Value"=w1578:u16)  [unwired: 2 in, 2 out]
                n620 = property on="C24" class="DigNum (strict)"() -> ("Value"=w1575:u16)  [unwired: 2 in, 2 out]
                n621 = Add(x=u16 1, y=w1578) -> (x+y=w1581:u16)
                n622 = Equal?(x=w1581, y=u16 1000) -> (x = y?=w1579:bool)
                n623 = Add(x=u16 1, y=w1576) -> (x+y=w1601:u16)
                n624 = Equal?(x=w1601, y=u16 1000) -> (x = y?=w1599:bool)
                n625 = Add(x=u16 1, y=w1577) -> (x+y=w1596:u16)
                n626 = Equal?(x=w1596, y=u16 1000) -> (x = y?=w1598:bool)
                n627 = Add(x=u16 1, y=w1575) -> (x+y=w1628:u16)
                n628 = Equal?(x=w1628, y=u16 1000) -> (x = y?=w1630:bool)
                n629 = To Word Integer(number=w1584) -> (16bit integer=w1583:i16)
                n630 = To Word Integer(number=w1604) -> (16bit integer=w1603:i16)
                n631 = To Word Integer(number=w1593) -> (16bit integer=w1594:i16)
                n632 = To Word Integer(number=w1625) -> (16bit integer=w1626:i16)
                n633 = case shown="1000" w1581 {
                  selector: w1581 -> [w1659 _]
                  frame 0, Default {
                    n634 = property on="C27" class="DigNum (strict)"("Value"=w1659) -> ()  [unwired: 2 in, 2 out]
                  }
                  frame 1000 {
                    n635 = property on="C27" class="DigNum (strict)"("Value"=0) -> ()  [unwired: 2 in, 2 out]
                  }
                }
                n636 = case shown="1000" w1601 {
                  selector: w1601 -> [w1687 _]
                  frame 0, Default {
                    n637 = property on="C25" class="DigNum (strict)"("Value"=w1687) -> ()  [unwired: 2 in, 2 out]
                  }
                  frame 1000 {
                    n638 = property on="C25" class="DigNum (strict)"("Value"=0) -> ()  [unwired: 2 in, 2 out]
                  }
                }
                n639 = case shown="1000" w1596 {
                  selector: w1596 -> [w1673 _]
                  frame 0, Default {
                    n640 = property on="C26" class="DigNum (strict)"("Value"=w1673) -> ()  [unwired: 2 in, 2 out]
                  }
                  frame 1000 {
                    n641 = property on="C26" class="DigNum (strict)"("Value"=0) -> ()  [unwired: 2 in, 2 out]
                  }
                }
                n642 = case shown="1000" w1628 {
                  selector: w1628 -> [w1701 _]
                  frame 0, Default {
                    n643 = property on="C24" class="DigNum (strict)"("Value"=w1701) -> ()  [unwired: 2 in, 2 out]
                  }
                  frame 1000 {
                    n644 = property on="C24" class="DigNum (strict)"("Value"=0) -> ()  [unwired: 2 in, 2 out]
                  }
                }
                n645 = local write "Ring 0"(FALSE ("Ring 0")) -> ()
                n646 = local write "Ring 3"(FALSE ("Ring 0")) -> ()
                n647 = local write "Ring 7"(FALSE ("Ring 0")) -> ()
                n648 = local write "Ring 4"(FALSE ("Ring 0")) -> ()
                n649 = local write "Ring 1"(FALSE ("Ring 0")) -> ()
                n650 = Replace Array Subset(array=w1566, new element=w1583, index=w1578) -> (w1570:i16[])
                n651 = Replace Array Subset(array=w1568, new element=w1603, index=w1576) -> (w1572:i16[])
                n652 = Replace Array Subset(array=w1567, new element=w1594, index=w1577) -> (w1571:i16[])
                n653 = Replace Array Subset(array=w1569, new element=w1626, index=w1575) -> (w1573:i16[])
                n654 = local write "Ring 5"(FALSE ("Ring 0")) -> ()
                n655 = local write "Ring 2"(FALSE ("Ring 0")) -> ()
                n656 = case shown="True" w1579 {
                  tunnel: w1570 -> [_ w1652]
                  frame False {
                  }
                  frame True {
                    n657 = To Double Precision Float(number=w1652) -> (double precision float=w1648:dbl[])
                    n658 = Add Array Elements(numeric array=w1648) -> (sum=w1650:dbl)
                    n659 = Divide(x=w1650, y=1000.0) -> (x/y=w1649:dbl)
                    n660 = call <vilib>:"Peak Detector.vi"("peaks/valleys"=enum32{"Peaks", "Valleys"}."Peaks", "threshold"=w1649, "X"=w1648) -> ("Amplitudes"=w1654:dbl[], "Locations"=→"Locations C27":dbl[])  [unwired: 4 in, 3 out]
                    n661 = Array Size(array=w1654) -> (size(s)=w1655:i32)
                    n662 = Greater Or Equal?(x=w1655, y=1) -> (x >= y?=w1653:bool)
                    "C27" <- w1653
                    n663 = case shown="True" w1653 {
                      tunnel: w1652 -> [_ w1658]
                      frame False {
                      }
                      frame True {
                        "Channel 27" <- w1658
                      }
                    }
                  }
                }
                n664 = case shown="True" w1599 {
                  tunnel: w1572 -> [_ w1680]
                  frame False {
                  }
                  frame True {
                    n665 = To Double Precision Float(number=w1680) -> (double precision float=w1676:dbl[])
                    n666 = Add Array Elements(numeric array=w1676) -> (sum=w1679:dbl)
                    n667 = Divide(x=w1679, y=1000.0) -> (x/y=w1677:dbl)
                    n668 = call <vilib>:"Peak Detector.vi"("peaks/valleys"=enum32{"Peaks", "Valleys"}."Peaks", "threshold"=w1677, "X"=w1676) -> ("Amplitudes"=w1682:dbl[], "Locations"=→"Locations 25":dbl[])  [unwired: 4 in, 3 out]
                    n669 = Array Size(array=w1682) -> (size(s)=w1683:i32)
                    n670 = Greater Or Equal?(x=w1683, y=1) -> (x >= y?=w1681:bool)
                    "C25" <- w1681
                    n671 = case shown="True" w1681 {
                      tunnel: w1680 -> [_ w1686]
                      frame False {
                      }
                      frame True {
                        "Channel 25" <- w1686
                      }
                    }
                  }
                }
                n672 = case shown="True" w1598 {
                  tunnel: w1571 -> [_ w1666]
                  frame False {
                  }
                  frame True {
                    n673 = To Double Precision Float(number=w1666) -> (double precision float=w1662:dbl[])
                    n674 = Add Array Elements(numeric array=w1662) -> (sum=w1664:dbl)
                    n675 = Divide(x=w1664, y=1000.0) -> (x/y=w1663:dbl)
                    n676 = call <vilib>:"Peak Detector.vi"("peaks/valleys"=enum32{"Peaks", "Valleys"}."Peaks", "threshold"=w1663, "X"=w1662) -> ("Amplitudes"=w1668:dbl[], "Locations"=→"Locations C26":dbl[])  [unwired: 4 in, 3 out]
                    n677 = Array Size(array=w1668) -> (size(s)=w1669:i32)
                    n678 = Greater Or Equal?(x=w1669, y=1) -> (x >= y?=w1667:bool)
                    "C26" <- w1667
                    n679 = case shown="True" w1667 {
                      tunnel: w1666 -> [_ w1672]
                      frame False {
                      }
                      frame True {
                        "Channel 26" <- w1672
                      }
                    }
                  }
                }
                n680 = case shown="True" w1630 {
                  tunnel: w1573 -> [_ w1694]
                  frame False {
                  }
                  frame True {
                    n681 = To Double Precision Float(number=w1694) -> (double precision float=w1690:dbl[])
                    n682 = Add Array Elements(numeric array=w1690) -> (sum=w1692:dbl)
                    n683 = Divide(x=w1692, y=1000.0) -> (x/y=w1691:dbl)
                    n684 = call <vilib>:"Peak Detector.vi"("peaks/valleys"=enum32{"Peaks", "Valleys"}."Peaks", "threshold"=w1691, "X"=w1690) -> ("Amplitudes"=w1696:dbl[], "Locations"=→"Locations C24":dbl[])  [unwired: 4 in, 3 out]
                    n685 = Array Size(array=w1696) -> (size(s)=w1697:i32)
                    n686 = Greater Or Equal?(x=w1697, y=1) -> (x >= y?=w1695:bool)
                    "C24" <- w1695
                    n687 = case shown="True" w1695 {
                      tunnel: w1694 -> [_ w1700]
                      frame False {
                      }
                      frame True {
                        "Channel 24" <- w1700
                      }
                    }
                  }
                }
                "Ring 6" <- TRUE ("Ring 6")
              }
              frame 28 {
                # "C31"
                # "C30"
                # "C29"
                # "C28"
                n688 = VISA Read(VISA resource name=w1794, byte count=u32 8, error in (no error)=w1793) -> (read buffer=w1756:string)  [unwired: 3 out]
                n689 = String To Byte Array(string=w1756) -> (unsigned byte array=w1724:u8[])
                n690 = Index Array(array=w1724, index=7) -> (element=w1734:u8)
                n691 = Index Array(array=w1724, index=6) -> (element=w1735:u8)
                n692 = Index Array(array=w1724, index=5) -> (element=w1737:u8)
                n693 = Index Array(array=w1724, index=4) -> (element=w1736:u8)
                n694 = Index Array(array=w1724, index=3) -> (element=w1750:u8)
                n695 = Index Array(array=w1724, index=2) -> (element=w1751:u8)
                n696 = Index Array(array=w1724, index=1) -> (element=w1758:u8)
                n697 = Index Array(array=w1724, index=0) -> (element=w1757:u8)
                n698 = Join Numbers(hi=w1734, lo=w1735) -> ((hi.lo)=w1733:u16)
                n699 = Join Numbers(hi=w1737, lo=w1736) -> ((hi.lo)=w1738:u16)
                n700 = Join Numbers(hi=w1750, lo=w1751) -> ((hi.lo)=w1749:u16)
                n701 = Join Numbers(hi=w1758, lo=w1757) -> ((hi.lo)=w1759:u16)
                n702 = property on="C29" class="DigNum (strict)"() -> ("Value"=w1727:u16)  [unwired: 2 in, 2 out]
                n703 = property on="C28" class="DigNum (strict)"() -> ("Value"=w1752:u16)  [unwired: 2 in, 2 out]
                n704 = property on="C30" class="DigNum (strict)"() -> ("Value"=w1726:u16)  [unwired: 2 in, 2 out]
                n705 = property on="C31" class="DigNum (strict)"() -> ("Value"=w1725:u16)  [unwired: 2 in, 2 out]
                n706 = local write "Ring 0"(FALSE ("Ring 0")) -> ()
                n707 = local write "Ring 3"(FALSE ("Ring 0")) -> ()
                n708 = Add(x=u16 1, y=w1725) -> (x+y=w1730:u16)
                n709 = Equal?(x=w1730, y=u16 1000) -> (x = y?=w1728:bool)
                n710 = Add(x=u16 1, y=w1726) -> (x+y=w1741:u16)
                n711 = Equal?(x=w1741, y=u16 1000) -> (x = y?=w1743:bool)
                n712 = Add(x=u16 1, y=w1727) -> (x+y=w1746:u16)
                n713 = Equal?(x=w1746, y=u16 1000) -> (x = y?=w1744:bool)
                n714 = Add(x=u16 1, y=w1752) -> (x+y=w1762:u16)
                n715 = Equal?(x=w1762, y=u16 1000) -> (x = y?=w1764:bool)
                n716 = To Word Integer(number=w1733) -> (16bit integer=w1732:i16)
                n717 = To Word Integer(number=w1738) -> (16bit integer=w1739:i16)
                n718 = To Word Integer(number=w1749) -> (16bit integer=w1748:i16)
                n719 = To Word Integer(number=w1759) -> (16bit integer=w1760:i16)
                n720 = case shown="1000" w1730 {
                  selector: w1730 -> [w1808 _]
                  frame 0, Default {
                    n721 = property on="C31" class="DigNum (strict)"("Value"=w1808) -> ()  [unwired: 2 in, 2 out]
                  }
                  frame 1000 {
                    n722 = property on="C31" class="DigNum (strict)"("Value"=0) -> ()  [unwired: 2 in, 2 out]
                  }
                }
                n723 = case shown="1000" w1741 {
                  selector: w1741 -> [w1822 _]
                  frame 0, Default {
                    n724 = property on="C30" class="DigNum (strict)"("Value"=w1822) -> ()  [unwired: 2 in, 2 out]
                  }
                  frame 1000 {
                    n725 = property on="C30" class="DigNum (strict)"("Value"=0) -> ()  [unwired: 2 in, 2 out]
                  }
                }
                n726 = case shown="1000" w1746 {
                  selector: w1746 -> [w1836 _]
                  frame 0, Default {
                    n727 = property on="C29" class="DigNum (strict)"("Value"=w1836) -> ()  [unwired: 2 in, 2 out]
                  }
                  frame 1000 {
                    n728 = property on="C29" class="DigNum (strict)"("Value"=0) -> ()  [unwired: 2 in, 2 out]
                  }
                }
                n729 = case shown="1000" w1762 {
                  selector: w1762 -> [w1850 _]
                  frame 0, Default {
                    n730 = property on="C28" class="DigNum (strict)"("Value"=w1850) -> ()  [unwired: 2 in, 2 out]
                  }
                  frame 1000 {
                    n731 = property on="C28" class="DigNum (strict)"("Value"=0) -> ()  [unwired: 2 in, 2 out]
                  }
                }
                n732 = local write "Ring 4"(FALSE ("Ring 0")) -> ()
                n733 = local write "Ring 1"(FALSE ("Ring 0")) -> ()
                n734 = local write "Ring 6"(FALSE ("Ring 0")) -> ()
                n735 = local write "Ring 5"(FALSE ("Ring 0")) -> ()
                n736 = local write "Ring 2"(FALSE ("Ring 0")) -> ()
                n737 = Replace Array Subset(array=w1711, new element=w1732, index=w1725) -> (w1712:i16[])
                n738 = Replace Array Subset(array=w1714, new element=w1739, index=w1726) -> (w1713:i16[])
                n739 = Replace Array Subset(array=w1716, new element=w1748, index=w1727) -> (w1715:i16[])
                n740 = Replace Array Subset(array=w1717, new element=w1760, index=w1752) -> (w1753:i16[])
                n741 = case shown="True" w1728 {
                  tunnel: w1712 -> [_ w1801]
                  frame False {
                  }
                  frame True {
                    n742 = To Double Precision Float(number=w1801) -> (double precision float=w1797:dbl[])
                    n743 = Add Array Elements(numeric array=w1797) -> (sum=w1799:dbl)
                    n744 = Divide(x=w1799, y=1000.0) -> (x/y=w1798:dbl)
                    n745 = call <vilib>:"Peak Detector.vi"("peaks/valleys"=enum32{"Peaks", "Valleys"}."Peaks", "threshold"=w1798, "X"=w1797) -> ("Amplitudes"=w1803:dbl[], "Locations"=→"Locations C31":dbl[])  [unwired: 4 in, 3 out]
                    n746 = Array Size(array=w1803) -> (size(s)=w1804:i32)
                    n747 = Greater Or Equal?(x=w1804, y=1) -> (x >= y?=w1802:bool)
                    "C31" <- w1802
                    n748 = case shown="True" w1802 {
                      tunnel: w1801 -> [_ w1807]
                      frame False {
                      }
                      frame True {
                        "Channel 31" <- w1807
                      }
                    }
                  }
                }
                n749 = case shown="True" w1743 {
                  tunnel: w1713 -> [_ w1815]
                  frame False {
                  }
                  frame True {
                    n750 = To Double Precision Float(number=w1815) -> (double precision float=w1811:dbl[])
                    n751 = Add Array Elements(numeric array=w1811) -> (sum=w1814:dbl)
                    n752 = Divide(x=w1814, y=1000.0) -> (x/y=w1812:dbl)
                    n753 = call <vilib>:"Peak Detector.vi"("peaks/valleys"=enum32{"Peaks", "Valleys"}."Peaks", "threshold"=w1812, "X"=w1811) -> ("Amplitudes"=w1817:dbl[], "Locations"=→"Locations C30":dbl[])  [unwired: 4 in, 3 out]
                    n754 = Array Size(array=w1817) -> (size(s)=w1818:i32)
                    n755 = Greater Or Equal?(x=w1818, y=1) -> (x >= y?=w1816:bool)
                    "C30" <- w1816
                    n756 = case shown="True" w1816 {
                      tunnel: w1815 -> [_ w1821]
                      frame False {
                      }
                      frame True {
                        "Channel 30" <- w1821
                      }
                    }
                  }
                }
                n757 = case shown="True" w1744 {
                  tunnel: w1715 -> [_ w1829]
                  frame False {
                  }
                  frame True {
                    n758 = To Double Precision Float(number=w1829) -> (double precision float=w1825:dbl[])
                    n759 = Add Array Elements(numeric array=w1825) -> (sum=w1827:dbl)
                    n760 = Divide(x=w1827, y=1000.0) -> (x/y=w1826:dbl)
                    n761 = call <vilib>:"Peak Detector.vi"("peaks/valleys"=enum32{"Peaks", "Valleys"}."Peaks", "threshold"=w1826, "X"=w1825) -> ("Amplitudes"=w1831:dbl[], "Locations"=→"Locations C29":dbl[])  [unwired: 4 in, 3 out]
                    n762 = Array Size(array=w1831) -> (size(s)=w1832:i32)
                    n763 = Greater Or Equal?(x=w1832, y=1) -> (x >= y?=w1830:bool)
                    "C29" <- w1830
                    n764 = case shown="True" w1830 {
                      tunnel: w1829 -> [_ w1835]
                      frame False {
                      }
                      frame True {
                        "Channel 29" <- w1835
                      }
                    }
                  }
                }
                n765 = case shown="True" w1764 {
                  tunnel: w1753 -> [_ w1843]
                  frame False {
                  }
                  frame True {
                    n766 = To Double Precision Float(number=w1843) -> (double precision float=w1839:dbl[])
                    n767 = Add Array Elements(numeric array=w1839) -> (sum=w1842:dbl)
                    n768 = Divide(x=w1842, y=1000.0) -> (x/y=w1840:dbl)
                    n769 = call <vilib>:"Peak Detector.vi"("peaks/valleys"=enum32{"Peaks", "Valleys"}."Peaks", "threshold"=w1840, "X"=w1839) -> ("Amplitudes"=w1845:dbl[], "Locations"=→"Locations 28":dbl[])  [unwired: 4 in, 3 out]
                    n770 = Array Size(array=w1845) -> (size(s)=w1846:i32)
                    n771 = Greater Or Equal?(x=w1846, y=1) -> (x >= y?=w1844:bool)
                    "C28" <- w1844
                    n772 = case shown="True" w1844 {
                      tunnel: w1843 -> [_ w1849]
                      frame False {
                      }
                      frame True {
                        "Channel 28" <- w1849
                      }
                    }
                  }
                }
                "Ring 7" <- TRUE ("Ring 7")
              }
              frame 1, Default {
              }
            }
          }
        }
      }
    }
    n773 = case shown="False" "?" {
      tunnel: w120 -> [_ w363]
      tunnel: w126 -> [_ w362]
      frame False {
      }
      frame True {
        n774 = Build Array(u8 1 ("element"), u8 4 ("element")) -> (w366:u8[])
        n775 = Byte Array To String(unsigned byte array=w366) -> (string=w365:string)
        n776 = VISA Write(VISA resource name=w362, write buffer=w365, error in (no error)=w363) -> ()  [unwired: 3 out]
        "?" <- TRUE ("Auto Stimulation")
      }
    }
    n777 = case shown="True" "Stimulate" {
      tunnel: w120 -> [_ w344]
      tunnel: w119 -> [_ w349]
      tunnel: "Infinite" -> [_ w348]
      tunnel: "Channel Number" -> [_ w273]
      frame False {
      }
      frame True {
        w268 = 0.0 ("y")
        w292 = 48000000
        w274 = 65536.0 ("y")
        w275 = 48.0 ("y")
        w276 = 24.0 ("y")
        # "Error Margin"
        # "Packet Size"
        # "# of cycles for 1 second"
        # "Stimulation Command Packet Type"
        n778 = case shown="False" w348 {
          tunnel: [w352 u16 65535] -> w347
          tunnel: "# of Stimulation\n       Cycles" -> [w352 _]
          frame False {
          }
          frame True {
          }
        }
        n779 = Multiply(x="Time 4", y=w292) -> (x*y=w271:dbl)
        n780 = Multiply(x="Time 2", y=w292) -> (x*y=w269:dbl)
        n781 = Multiply(x="Time 3", y=w292) -> (x*y=w267:dbl)
        n782 = Subtract(x=w271, y=w268) -> (x-y=w272:dbl)
        n783 = Subtract(x=w269, y=w268) -> (x-y=w270:dbl)
        n784 = Subtract(x=w267, y=w268) -> (x-y=w266:dbl)
        n785 = Add(x="Value 3", y=w276) -> (x+y=w310:dbl)
        n786 = Add(x="Value 2", y=w276) -> (x+y=w307:dbl)
        n787 = Add(x="Value", y=w276) -> (x+y=w283:dbl)
        n788 = Add(x="Value 4", y=w276) -> (x+y=w313:dbl)
        n789 = Multiply(x="Time", y=w292) -> (x*y=w291:dbl)
        n790 = Divide(x=w310, y=w275) -> (x/y=w309:dbl)
        n791 = Divide(x=w307, y=w275) -> (x/y=w306:dbl)
        n792 = Divide(x=w283, y=w275) -> (x/y=w282:dbl)
        n793 = Divide(x=w313, y=w275) -> (x/y=w312:dbl)
        n794 = Multiply(x=w309, y=w274) -> (x*y=w308:dbl)
        n795 = Multiply(x=w306, y=w274) -> (x*y=w305:dbl)
        n796 = Multiply(x=w282, y=w274) -> (x*y=w281:dbl)
        n797 = Multiply(x=w312, y=w274) -> (x*y=w311:dbl)
        n798 = To Long Integer(number=w272) -> (32bit integer=w340:i32)
        n799 = To Long Integer(number=w270) -> (32bit integer=w335:i32)
        n800 = To Long Integer(number=w291) -> (32bit integer=w290:i32)
        n801 = To Long Integer(number=w266) -> (32bit integer=w332:i32)
        n802 = To Unsigned Word Integer(number=w308) -> (unsigned 16bit integer=w342:u16)
        n803 = To Unsigned Word Integer(number=w305) -> (unsigned 16bit integer=w341:u16)
        n804 = To Unsigned Word Integer(number=w281) -> (unsigned 16bit integer=w279:u16)
        n805 = To Unsigned Word Integer(number=w311) -> (unsigned 16bit integer=w343:u16)
        n806 = Split Number(x=w340) -> (hi(x)=w339:u16, lo(x)=w338:u16)
        n807 = Split Number(x=w335) -> (hi(x)=w337:u16, lo(x)=w336:u16)
        n808 = Split Number(x=w290) -> (hi(x)=w288:u16, lo(x)=w289:u16)
        n809 = Split Number(x=w332) -> (hi(x)=w334:u16, lo(x)=w333:u16)
        n810 = Split Number(x=w339) -> (hi(x)=w328:u8, lo(x)=w329:u8)
        n811 = Split Number(x=w338) -> (hi(x)=w330:u8, lo(x)=w331:u8)
        n812 = Split Number(x=w337) -> (hi(x)=w322:u8, lo(x)=w323:u8)
        n813 = Split Number(x=w336) -> (hi(x)=w324:u8, lo(x)=w325:u8)
        n814 = Split Number(x="# of Pulse \n  Cycles") -> (hi(x)=w302:u8, lo(x)=w303:u8)
        n815 = Split Number(x=w288) -> (hi(x)=w284:u8, lo(x)=w285:u8)
        n816 = Split Number(x=w289) -> (hi(x)=w286:u8, lo(x)=w287:u8)
        n817 = Split Number(x=w334) -> (hi(x)=w316:u8, lo(x)=w317:u8)
        n818 = Split Number(x=w333) -> (hi(x)=w318:u8, lo(x)=w319:u8)
        n819 = Split Number(x=w342) -> (hi(x)=w320:u8, lo(x)=w321:u8)
        n820 = Split Number(x=w341) -> (hi(x)=w314:u8, lo(x)=w315:u8)
        n821 = Split Number(x=w279) -> (hi(x)=w277:u8, lo(x)=w278:u8)
        n822 = Split Number(x=w343) -> (hi(x)=w326:u8, lo(x)=w327:u8)
        n823 = Split Number(x=w347) -> (hi(x)=w345:u8, lo(x)=w346:u8)
        n824 = Build Array(u8 30 ("element"), u8 1 ("element"), w346, w345, w331, w330, w329, w328, w327, w326, w325, w324, w323, w322, w321, w320, w319, w318, w317, w316, w315, w314, w303, w302, w287, w286, w285, w284, w278, w277, w273) -> (w351:u8[])
        n825 = Byte Array To String(unsigned byte array=w351) -> (string=w350:string)
        n826 = VISA Write(VISA resource name=w349, write buffer=w350, error in (no error)=w344) -> ()  [unwired: 3 out]
      }
    }
    n827 = case shown="False" "Stop Stimulation" {
      tunnel: w119 -> [_ w360]
      tunnel: w120 -> [_ w359]
      tunnel: "Channel Number" -> [_ w355]
      frame False {
      }
      frame True {
        # "Packet Size"
        # "Stop Stimulation Packet Data Type"
        n828 = Build Array(u8 2 ("element"), u8 2 ("element"), w355) -> (w357:u8[])
        n829 = Byte Array To String(unsigned byte array=w357) -> (string=w356:string)
        n830 = VISA Write(VISA resource name=w360, write buffer=w356, error in (no error)=w359) -> ()  [unwired: 3 out]
      }
    }
    n831 = case shown="True" "?" {
      frame False {
      }
      frame True {
        n832 = case shown="\"CHANNEL 0\", Default" "Select Channel" {
          tunnel: [w233 w234 w235 w236 w237 w238 w239 w240 w241 w242 w243 w244 w245 w246 w247 w248 w249 w250 w251 w252 w253 w254 w255 w256 w257 w258 w259 w260 w261 w262 w263 w264] -> w196
          frame "CHANNEL 0", Default {
            n833 = property on="Locations C0" class="Arr (strict)"() -> ("Value"=w233:dbl[])  [unwired: 2 in, 2 out]
          }
          frame "CHANNEL 1" {
            n834 = property on="Locations C1" class="Arr (strict)"() -> ("Value"=w234:dbl[])  [unwired: 2 in, 2 out]
          }
          frame "CHANNEL 2 " {
            n835 = property on="Locations C2" class="Arr (strict)"() -> ("Value"=w235:dbl[])  [unwired: 2 in, 2 out]
          }
          frame "CHANNEL 3 " {
            n836 = property on="Locations C3" class="Arr (strict)"() -> ("Value"=w236:dbl[])  [unwired: 2 in, 2 out]
          }
          frame "CHANNEL 4 " {
            n837 = property on="Locations C4" class="Arr (strict)"() -> ("Value"=w237:dbl[])  [unwired: 2 in, 2 out]
          }
          frame "CHANNEL 5 " {
            n838 = property on="Locations C5" class="Arr (strict)"() -> ("Value"=w238:dbl[])  [unwired: 2 in, 2 out]
          }
          frame "CHANNEL 6" {
            n839 = property on="Locations C6" class="Arr (strict)"() -> ("Value"=w239:dbl[])  [unwired: 2 in, 2 out]
          }
          frame "CHANNEL  7" {
            n840 = property on="Locations C7" class="Arr (strict)"() -> ("Value"=w240:dbl[])  [unwired: 2 in, 2 out]
          }
          frame "CHANNEL 8 " {
            n841 = property on="Locations C8" class="Arr (strict)"() -> ("Value"=w241:dbl[])  [unwired: 2 in, 2 out]
          }
          frame "CHANNEL 9" {
            n842 = property on="Locations C9" class="Arr (strict)"() -> ("Value"=w242:dbl[])  [unwired: 2 in, 2 out]
          }
          frame "CHANNEL 10" {
            n843 = property on="Locations C10" class="Arr (strict)"() -> ("Value"=w243:dbl[])  [unwired: 2 in, 2 out]
          }
          frame "CHANNEL 11" {
            n844 = property on="Locations C11" class="Arr (strict)"() -> ("Value"=w244:dbl[])  [unwired: 2 in, 2 out]
          }
          frame "CHANNEL 12" {
            n845 = property on="Locations 12" class="Arr (strict)"() -> ("Value"=w245:dbl[])  [unwired: 2 in, 2 out]
          }
          frame "CHANNEL 13" {
            n846 = property on="Locations 13" class="Arr (strict)"() -> ("Value"=w246:dbl[])  [unwired: 2 in, 2 out]
          }
          frame "CHANNEL 14" {
            n847 = property on="Locations C14" class="Arr (strict)"() -> ("Value"=w247:dbl[])  [unwired: 2 in, 2 out]
          }
          frame "CHANNEL 15" {
            n848 = property on="Locations C15" class="Arr (strict)"() -> ("Value"=w248:dbl[])  [unwired: 2 in, 2 out]
          }
          frame "CHANNEL 16" {
            n849 = property on="Locations C16" class="Arr (strict)"() -> ("Value"=w249:dbl[])  [unwired: 2 in, 2 out]
          }
          frame "CHANNEL 17" {
            n850 = property on="Locations C17" class="Arr (strict)"() -> ("Value"=w250:dbl[])  [unwired: 2 in, 2 out]
          }
          frame "CHANNEL 18" {
            n851 = property on="Locations C18" class="Arr (strict)"() -> ("Value"=w251:dbl[])  [unwired: 2 in, 2 out]
          }
          frame "CHANNEL 19" {
            n852 = property on="Locations C19" class="Arr (strict)"() -> ("Value"=w252:dbl[])  [unwired: 2 in, 2 out]
          }
          frame "CHANNEL 20" {
            n853 = property on="Locations C20" class="Arr (strict)"() -> ("Value"=w253:dbl[])  [unwired: 2 in, 2 out]
          }
          frame "CHANNEL 21" {
            n854 = property on="Locations C21" class="Arr (strict)"() -> ("Value"=w254:dbl[])  [unwired: 2 in, 2 out]
          }
          frame "CHANNEL 22" {
            n855 = property on="Locations C22" class="Arr (strict)"() -> ("Value"=w255:dbl[])  [unwired: 2 in, 2 out]
          }
          frame "CHANNEL 23" {
            n856 = property on="Locations C23" class="Arr (strict)"() -> ("Value"=w256:dbl[])  [unwired: 2 in, 2 out]
          }
          frame "CHANNEL 24" {
            n857 = property on="Locations C24" class="Arr (strict)"() -> ("Value"=w257:dbl[])  [unwired: 2 in, 2 out]
          }
          frame "CHANNEL 25" {
            n858 = property on="Locations 25" class="Arr (strict)"() -> ("Value"=w258:dbl[])  [unwired: 2 in, 2 out]
          }
          frame "CHANNEL 26" {
            n859 = property on="Locations C26" class="Arr (strict)"() -> ("Value"=w259:dbl[])  [unwired: 2 in, 2 out]
          }
          frame "CHANNEL 27" {
            n860 = property on="Locations C27" class="Arr (strict)"() -> ("Value"=w260:dbl[])  [unwired: 2 in, 2 out]
          }
          frame "CHANNEL 28" {
            n861 = property on="Locations 28" class="Arr (strict)"() -> ("Value"=w261:dbl[])  [unwired: 2 in, 2 out]
          }
          frame "CHANNEL 29" {
            n862 = property on="Locations C29" class="Arr (strict)"() -> ("Value"=w262:dbl[])  [unwired: 2 in, 2 out]
          }
          frame "CHANNEL 30" {
            n863 = property on="Locations C30" class="Arr (strict)"() -> ("Value"=w263:dbl[])  [unwired: 2 in, 2 out]
          }
          frame "CHANNEL 31" {
            n864 = property on="Locations C31" class="Arr (strict)"() -> ("Value"=w264:dbl[])  [unwired: 2 in, 2 out]
          }
        }
        n865 = case shown="\"CHANNEL 4 \"" "Select Channel 2" {
          tunnel: [w201 w202 w203 w204 w205 w206 w207 w208 w209 w210 w211 w212 w213 w214 w215 w216 w217 w218 w219 w220 w221 w222 w223 w224 w225 w226 w227 w228 w229 w230 w231 w232] -> w197
          frame "CHANNEL 0", Default {
            n866 = property on="Locations C0" class="Arr (strict)"() -> ("Value"=w201:dbl[])  [unwired: 2 in, 2 out]
          }
          frame "CHANNEL 1" {
            n867 = property on="Locations C1" class="Arr (strict)"() -> ("Value"=w202:dbl[])  [unwired: 2 in, 2 out]
          }
          frame "CHANNEL 2 " {
            n868 = property on="Locations C2" class="Arr (strict)"() -> ("Value"=w203:dbl[])  [unwired: 2 in, 2 out]
          }
          frame "CHANNEL 3 " {
            n869 = property on="Locations C3" class="Arr (strict)"() -> ("Value"=w204:dbl[])  [unwired: 2 in, 2 out]
          }
          frame "CHANNEL 4 " {
            n870 = property on="Locations C4" class="Arr (strict)"() -> ("Value"=w205:dbl[])  [unwired: 2 in, 2 out]
          }
          frame "CHANNEL 5 " {
            n871 = property on="Locations C5" class="Arr (strict)"() -> ("Value"=w206:dbl[])  [unwired: 2 in, 2 out]
          }
          frame "CHANNEL 6" {
            n872 = property on="Locations C6" class="Arr (strict)"() -> ("Value"=w207:dbl[])  [unwired: 2 in, 2 out]
          }
          frame "CHANNEL  7" {
            n873 = property on="Locations C7" class="Arr (strict)"() -> ("Value"=w208:dbl[])  [unwired: 2 in, 2 out]
          }
          frame "CHANNEL 8 " {
            n874 = property on="Locations C8" class="Arr (strict)"() -> ("Value"=w209:dbl[])  [unwired: 2 in, 2 out]
          }
          frame "CHANNEL 9" {
            n875 = property on="Locations C9" class="Arr (strict)"() -> ("Value"=w210:dbl[])  [unwired: 2 in, 2 out]
          }
          frame "CHANNEL 10" {
            n876 = property on="Locations C10" class="Arr (strict)"() -> ("Value"=w211:dbl[])  [unwired: 2 in, 2 out]
          }
          frame "CHANNEL 11" {
            n877 = property on="Locations C11" class="Arr (strict)"() -> ("Value"=w212:dbl[])  [unwired: 2 in, 2 out]
          }
          frame "CHANNEL 12" {
            n878 = property on="Locations 12" class="Arr (strict)"() -> ("Value"=w213:dbl[])  [unwired: 2 in, 2 out]
          }
          frame "CHANNEL 13" {
            n879 = property on="Locations 13" class="Arr (strict)"() -> ("Value"=w214:dbl[])  [unwired: 2 in, 2 out]
          }
          frame "CHANNEL 14" {
            n880 = property on="Locations C14" class="Arr (strict)"() -> ("Value"=w215:dbl[])  [unwired: 2 in, 2 out]
          }
          frame "CHANNEL 15" {
            n881 = property on="Locations C15" class="Arr (strict)"() -> ("Value"=w216:dbl[])  [unwired: 2 in, 2 out]
          }
          frame "CHANNEL 16" {
            n882 = property on="Locations C16" class="Arr (strict)"() -> ("Value"=w217:dbl[])  [unwired: 2 in, 2 out]
          }
          frame "CHANNEL 17" {
            n883 = property on="Locations C17" class="Arr (strict)"() -> ("Value"=w218:dbl[])  [unwired: 2 in, 2 out]
          }
          frame "CHANNEL 18" {
            n884 = property on="Locations C18" class="Arr (strict)"() -> ("Value"=w219:dbl[])  [unwired: 2 in, 2 out]
          }
          frame "CHANNEL 19" {
            n885 = property on="Locations C19" class="Arr (strict)"() -> ("Value"=w220:dbl[])  [unwired: 2 in, 2 out]
          }
          frame "CHANNEL 20" {
            n886 = property on="Locations C20" class="Arr (strict)"() -> ("Value"=w221:dbl[])  [unwired: 2 in, 2 out]
          }
          frame "CHANNEL 21" {
            n887 = property on="Locations C21" class="Arr (strict)"() -> ("Value"=w222:dbl[])  [unwired: 2 in, 2 out]
          }
          frame "CHANNEL 22" {
            n888 = property on="Locations C22" class="Arr (strict)"() -> ("Value"=w223:dbl[])  [unwired: 2 in, 2 out]
          }
          frame "CHANNEL 23" {
            n889 = property on="Locations C23" class="Arr (strict)"() -> ("Value"=w224:dbl[])  [unwired: 2 in, 2 out]
          }
          frame "CHANNEL 24" {
            n890 = property on="Locations C24" class="Arr (strict)"() -> ("Value"=w225:dbl[])  [unwired: 2 in, 2 out]
          }
          frame "CHANNEL 25" {
            n891 = property on="Locations 25" class="Arr (strict)"() -> ("Value"=w226:dbl[])  [unwired: 2 in, 2 out]
          }
          frame "CHANNEL 26" {
            n892 = property on="Locations C26" class="Arr (strict)"() -> ("Value"=w227:dbl[])  [unwired: 2 in, 2 out]
          }
          frame "CHANNEL 27" {
            n893 = property on="Locations C27" class="Arr (strict)"() -> ("Value"=w228:dbl[])  [unwired: 2 in, 2 out]
          }
          frame "CHANNEL 28" {
            n894 = property on="Locations 28" class="Arr (strict)"() -> ("Value"=w229:dbl[])  [unwired: 2 in, 2 out]
          }
          frame "CHANNEL 29" {
            n895 = property on="Locations C29" class="Arr (strict)"() -> ("Value"=w230:dbl[])  [unwired: 2 in, 2 out]
          }
          frame "CHANNEL 30" {
            n896 = property on="Locations C30" class="Arr (strict)"() -> ("Value"=w231:dbl[])  [unwired: 2 in, 2 out]
          }
          frame "CHANNEL 31" {
            n897 = property on="Locations C31" class="Arr (strict)"() -> ("Value"=w232:dbl[])  [unwired: 2 in, 2 out]
          }
        }
        n898 = Subtract(x=w196, y=w197) -> (x-y=→"DIFFERENCE":dbl[])
      }
    }
    n899 = property on="C0 index position" class="DigNum (strict)"() -> ("Value"=w110:i32)  [unwired: 2 in, 2 out]
    n900 = property on="Ch4 index position" class="DigNum (strict)"() -> ("Value"=w109:i32)  [unwired: 2 in, 2 out]
    n901 = property on="C4  max value" class="DigNum (strict)"() -> ("Value"=w114:dbl)  [unwired: 2 in, 2 out]
    n902 = property on="C0 max value" class="DigNum (strict)"() -> ("Value"=w113:dbl)  [unwired: 2 in, 2 out]
    n903 = Subtract(x=w114, y=w113) -> (x-y=→"max difference":dbl)
    n904 = Subtract(x=w109, y=w110) -> (x-y=→"Difference Index":i32)
    n905 = Unbundle By Name(w120) -> ("status"=w191:bool)
  }
  n906 = VISA Close(VISA resource name=w99, error in (no error)=w98) -> ()  [unwired: 1 out]
  n907 = property on="Locations C1" class="Arr (strict)" props=["Value"]() -> ()  [unwired: 2 in, 3 out]
  n908 = property on="Locations C0" class="Arr (strict)" props=["Value"]() -> ()  [unwired: 2 in, 3 out]
  n909 = property on="Locations C2" class="Arr (strict)" props=["Value"]() -> ()  [unwired: 2 in, 3 out]
  n910 = property on="Locations C3" class="Arr (strict)" props=["Value"]() -> ()  [unwired: 2 in, 3 out]
  n911 = property on="Locations C4" class="Arr (strict)" props=["Value"]() -> ()  [unwired: 2 in, 3 out]
  n912 = property on="Locations C6" class="Arr (strict)" props=["Value"]() -> ()  [unwired: 2 in, 3 out]
  n913 = property on="Locations C7" class="Arr (strict)" props=["Value"]() -> ()  [unwired: 2 in, 3 out]
  n914 = property on="Locations C5" class="Arr (strict)" props=["Value"]() -> ()  [unwired: 2 in, 3 out]
  n915 = property on="Locations C8" class="Arr (strict)" props=["Value"]() -> ()  [unwired: 2 in, 3 out]
  n916 = property on="Locations C9" class="Arr (strict)" props=["Value"]() -> ()  [unwired: 2 in, 3 out]
  n917 = property on="Locations C10" class="Arr (strict)" props=["Value"]() -> ()  [unwired: 2 in, 3 out]
  n918 = property on="Locations C11" class="Arr (strict)" props=["Value"]() -> ()  [unwired: 2 in, 3 out]
  n919 = property on="Locations C15" class="Arr (strict)" props=["Value"]() -> ()  [unwired: 2 in, 3 out]
  n920 = property on="Locations C14" class="Arr (strict)" props=["Value"]() -> ()  [unwired: 2 in, 3 out]
  n921 = property on="Locations 12" class="Arr (strict)" props=["Value"]() -> ()  [unwired: 2 in, 3 out]
  n922 = property on="Locations 13" class="Arr (strict)" props=["Value"]() -> ()  [unwired: 2 in, 3 out]
  n923 = property on="Locations C19" class="Arr (strict)" props=["Value"]() -> ()  [unwired: 2 in, 3 out]
  n924 = property on="Locations C18" class="Arr (strict)" props=["Value"]() -> ()  [unwired: 2 in, 3 out]
  n925 = property on="Locations C16" class="Arr (strict)" props=["Value"]() -> ()  [unwired: 2 in, 3 out]
  n926 = property on="Locations C17" class="Arr (strict)" props=["Value"]() -> ()  [unwired: 2 in, 3 out]
  n927 = property on="Locations C23" class="Arr (strict)" props=["Value"]() -> ()  [unwired: 2 in, 3 out]
  n928 = property on="Locations C21" class="Arr (strict)" props=["Value"]() -> ()  [unwired: 2 in, 3 out]
  n929 = property on="Locations C20" class="Arr (strict)" props=["Value"]() -> ()  [unwired: 2 in, 3 out]
  n930 = property on="Locations C22" class="Arr (strict)" props=["Value"]() -> ()  [unwired: 2 in, 3 out]
  n931 = property on="Locations C24" class="Arr (strict)" props=["Value"]() -> ()  [unwired: 2 in, 3 out]
  n932 = property on="Locations 25" class="Arr (strict)" props=["Value"]() -> ()  [unwired: 2 in, 3 out]
  n933 = property on="Locations C26" class="Arr (strict)" props=["Value"]() -> ()  [unwired: 2 in, 3 out]
  n934 = property on="Locations C27" class="Arr (strict)" props=["Value"]() -> ()  [unwired: 2 in, 3 out]
  n935 = property on="Locations 28" class="Arr (strict)" props=["Value"]() -> ()  [unwired: 2 in, 3 out]
  n936 = property on="Locations C29" class="Arr (strict)" props=["Value"]() -> ()  [unwired: 2 in, 3 out]
  n937 = property on="Locations C30" class="Arr (strict)" props=["Value"]() -> ()  [unwired: 2 in, 3 out]
  n938 = property on="Locations C31" class="Arr (strict)" props=["Value"]() -> ()  [unwired: 2 in, 3 out]
